vi "UHR-Fleezers Control (fpga) - avogadro 2.vi"() -> ()   [LabVIEW 2014]
doc: "UHR-Fleezers Instrument Control Code (fpga)"
uses:
  <vilib>/Platform/TimedLoop/XDataNode/timing_clust.ctl
  <vilib>/Platform/TimedLoop/XDataNode/nitl_modes.ctl
  <vilib>/Platform/TimedLoop/XDataNode/wakeup.ctl
  <vilib>/rvi/Emulation/niFpgaGetClockAttributes.vi
  <vilib>/rvi/Emulation/niFpgaSctlEmulationGetInTimedLoop.vi
  <vilib>/rvi/Emulation/niFpgaEmulationReportErrorSimple.vi
  <vilib>/rvi/Emulation/niFpgaProcessEmulError.vi
  <vilib>/rvi/eio/common/nirviEmuTemplateMethod_errors.vi
  <vilib>/rvi/interface/RandomDataEmulation/niFpgaRandomDataHandleErrors.vi
  <vilib>/rvi/Emulation/niFpgaCriticalErrorInLSC.vi
  <vilib>/eio/EIONode/EIONode.xnode
  <vilib>/eio/EIOMethodNode/EIOMethodNode.xnode
  <vilib>/rvi/DataTransferAndStorage/Container/XNode/niFpgaContainer.xnode
  <vilib>/rvi/interface/RandomDataEmulation/nirviRandomDataFpgaReadWriteTemplate.vi
  <vilib>/addons/control/pid/fpga.llb/XNode/niFpgaPID.xnode
  <vilib>/Platform/TimedLoop/XDataNode/XDataNode.xnode
  <vilib>/Platform/TimedLoop/XDataNode/XDNodeRunTimeDep.lvlib
panel:
  out "Tab Control":T1(tab)=enum."MCL trap control"
  in  "Set 3":bool
  in  "Set 2":bool=TRUE
  in  "Set 1":bool=TRUE
  in  "Trap Pos to FIFO":bool
  in  "N of AI1 Int Acq Sets":i16=2 min=1 max=3 step=1
  out "AI Late Counter":u8
  in  "ai count":u16=400
  in  "+ phase":bool
  in  "Phase count adjustment":i16
  out "Relative phase":i16
  in  "AI to FIFO":bool
  out "BD1 Frequency Out 1":u64
  out "BD1 Frequency Out 2":u64
  out "Trap Pos FIFO Timeout":u16
  out "Trap AI FIFO Timeout":u16
  in  "Trap FIFO Set Timeout":i32
  out "Tab Control 2":T2(tab)
  in  "Piezo offset Y points":u64
  in  "Piezo offset X points":u64
  in  "Piezo offset Xmin":u64
  in  "Piezo Offset Ymin":u64
  in  "Piezo Offset Increment":u64
  in  "Multiple trap 3 position offset \nfile":bool
  in  "FB output range":cluster{"output low":i16, "output high":i16}={"output low"=0, "output high"=3000}
  in  "FB Gains":T3={"proportional gain (Kc)"=10, "integral gain (Kc*Ts/Ti)"=5, "derivative gain (Kc*Td/Ts)"=0}
  in  "RD":bool
  in  "Swap F1 and F2":bool
  in  "Cont. Scan":bool
  in  "Abort scan":bool
  in  "Cycles per step":u64
  in  "Scan BD":bool
  in  "Number of scans":u16
  in  "Scan steps":u64
  in  "Scan freq.  increment":i64
  out "Scanning":bool
  in  "Start scan":bool
  in  "OSK Bd 1":bool
  in  "Reset Bd 1":bool
  in  "PMODE":bool
  in  "Direct RF Box \nCommunication":bool
  in  "Data BD 2":u8 format="%08b"
  in  "Data BD 1":u8 format="%08b"
  in  "Address":u8 format="%02x"
  in  "Update Data":bool
  in  "FPGA Controls\n RF Box":bool
  in  "Number Interlace Cycles":u8=2 min=1 max=3
  in  "Interlace Off Parameters":u8=1 min=1 max=3
  in  "Interlace ON/OFF":bool
  out "DIO Relative phase":i16
  in  "Phase count adjustment (DIO)":i16
  in  "+ phase (DIO)":bool
  out "DIO Late Counter":u8
  in  "DIO count 1 (ticks)":u16=400
  in  "DIO count 2 (ticks)":u16=400
  in  "DIO count 3 (ticks)":u16=400
  out "AI2 Y Sum Set 2":i16
  out "AI2 Y Sum Set 1":i16
  in  "FB Setpoint Set 1":i16 min=0 step=1
  in  "FB Reset Set 1":bool
  in  "FB On/Off Set 1":bool
  in  "FB Reset Set 2":bool
  in  "FB On/Off Set 2":bool
  in  "FB Setpoint Set 2":i16 min=0 step=1
  out "Scan I":u64
  in  "Amp switch delay":u8=5
  in  "BD 2 Amplitude 1":u16
  in  "BD 1 Amplitude 1":u16
  in  "BD 2 Frequency 1":u64
  in  "BD 1 Frequency 1":u64
  in  "BD 2 Amplitude 2":u16
  in  "BD 1 Amplitude 2":u16
  in  "BD 2 Frequency 2":u64
  in  "BD 1 Frequency 2":u64
  in  "BD 2 Amplitude 3":u16
  in  "BD 1 Amplitude 3":u16
  in  "BD 2 Frequency 3":u64
  in  "BD 1 Frequency 3":u64
  in  "BD 1 Delay (ticks)":u8
  in  "BD 2 Delay (Ticks)":u8 caption="Count(Ticks)"
  in  "Next trap write delay (ticks)":u8 caption="Count(Ticks)"
  out "Piezo X out":i16
  out "Piezo Y out":i16
  in  "Piezo Trap ON/Off (AO3)":i16
  in  "Piezo Trap X (AO5)":i16
  in  "Piezo Trap Y (AO4)":i16
  in  "Trap pos. FB Range":T4={"FB2 output low"=-1.0, "FB2 output high"=0.999969482421875}
  in  "FB Min frequency":u64
  in  "FB Max Frequency":u64
  in  "Dynamic Force FB (Ronen)":bool
  in  "Negate Diff?":bool
  in  "Diff FB Measurement?":bool
  in  "FB Trig Integrate":u32=1
  out "TTrig?":bool
  in  "TTrig Negate Pos":bool=TRUE
  out "Trap Pos FB Int Signal":fxp<+/-,24,9> format="%.18g"
  out "Trap Pos FB Int-Norm Signal":fxp<+/-,16,1> format="%.16g"
  in  "FPGA TTrig Thresh":i64
  in  "FPGA Trap Trig":bool
  out "Trap Pos FB Action":i64
  in  "Trap Pos. FB Offset Factor":i64
  in  "Trap Pos. FB Mult Factor":i64=2
  in  "Trap Pos. FB Reset":bool
  in  "Trap Pos FB Monitor T1 or T2":bool
  in  "AI1 X Scale":u16
  in  "Trap Pos FB Int Count":u16=100
  in  "Trap Pos FB Negate Action":bool
  out "AI1 X Set 2":fxp<+/-,16,1>
  out "AI1 X Set 1":fxp<+/-,16,1>
  in  "Trap Pos. FB SP":fxp<+/-,16,1>
  in  "Force feedback":bool
  out "TTrig Sig":i64
  out "TTrig Fin Thresh":i64
  in  "B factor":fxp<+/-,32,16>
  in  "Trap Pos. FB Gains":T5={"proportional gain (Kc)"=0.999969482421875, "integral gain (Kc*Ts/Ti)"=0.999969482421875, "derivative gain (Kc*Td/Ts)"=0.0}
  in  "ScanTrap 3 or Fl-laser":bool
  in  "1D or 2D Scan?":bool
  in  "Abort scan (MCL)":bool
  in  "MCL Scan Axis":bool
  in  "Cont. Scan (MCL)":bool
  out "Scan I (MCL)":u64
  in  "Number of scans (MCL)":u16
  out "Scanning MCL":bool
  in  "Scan steps (MCL)":u64
  in  "Cycles per step (MCL)":u64
  in  "Scan freq.  increment (MCL)":i16
  in  "Start scan (MCL)":bool
  in  "AO2 (X)":i16
  in  "AO1 (Y)":i16
  out "MCL Late Counter":u8
  in  "MCL count":u32=800
  out "MCL Relative Phase":i16
  in  "Phase count adjustment (MCL)":i16
  in  "+ phase (MCL)":bool
  out "APD2 int gate":bool
  out "APD3 out state":bool
  in  "APD Gate Operating Mode":u8 max=2 step=1
  in  "Invert APD Gate":bool
  in  "APD Gate OFF Count":u16=100
  in  "APD Gate ON Count":u16=300
  out "APD 1 Gate Late Counter":u8
  out "APD 1 Gate Relative Phase":i16
  in  "Phase count adjustment (APD 1 Gate)":i16
  in  "+ phase (APD 1 Gate)":bool
  out "APD 2 Counts 0":u32
  out "APD 2 Counts 1":u32
  out "APD 1 Counts 0":u32
  out "APD 1 Counts 1":u32
  out "APD1 out state":bool
  in  "APD AO scale factor":i16=1
  in  "APD to FIFO":bool
  in  "APD Acq Rate Count":u32=20000000
  out "APD Acq Late Counter":u8
  out "APD Acq Relative Phase":i16
  in  "Phase Count Adjustment (APD Acq)":i16
  in  "+ phase (APD Acq)":bool
  in  "Phase count adjustment (APD 2 Gate)":i16
  out "APD 2 Gate Late Counter":u8
  out "APD 2 Gate Relative Phase":i16
  in  "+ phase (APD 2 Gate)":bool
  out "APD2 out state":bool
  out "APD 3 Counts 0":u32
  out "APD 3 Counts 1":u32
  out "APD 3 Gate Late Counter":u8
  in  "Phase count adjustment (APD 3 Gate)":i16
  out "APD 3 Gate Relative Phase":i16
  in  "+ phase (APD 3 Gate)":bool
  out "APD1 int gate":bool
  out "APD3 int gate":bool
  in  "D3":i16
  in  "I3":i16=5
  in  "P3":i16=10
  in  "Green Filter Flipper":bool
  in  "Green FB Count":u16=1200
  out "Green Late Counter":u8
  out "Green FB Relative Phase":i16
  in  "Phase count adjustment (Green FB)":i16=10
  in  "+ phase (Green FB)":bool
  out "Green FB Sum":i16
  in  "Green int current ON count adj":u16=150
  in  "Current Out":u16=30000
  in  "Green FB On/Off":bool
  in  "Green FB Setpoint":i16=250 min=0 step=1
  in  "Green FB Reset":bool
  in  "Operating Mode 2":u8=2 max=2 step=1
  in  "Invert GI 2":bool
  in  "Green interlace OFF count 2":u16=900
  in  "Green interlace ON count 2":u16=300
  out "GI Late Counter 2":u8
  out "GI Relative phase 2":i16
  in  "Phase count adjustment (GI) 2":i16=20
  in  "+ phase (GI) 2":bool
  in  "Green interlace OFF count":u16=100
  out "GI Relative phase":i16
  in  "Phase count adjustment (GI)":i16
  in  "+ phase (GI)":bool
  in  "Green interlace ON count":u16=300
  out "GI Late Counter":u8
  in  "Invert GI":bool
  in  "Operating Mode":u8 max=2 step=1
  in  "+ phase (RI)":bool
  out "RI Relative phase":i16
  out "RI Late Counter":u8
  in  "Red interlace ON count":u16=300
  in  "Red interlace OFF count":u16=100
  in  "Invert RI":bool
  in  "Red Laser Operating Mode":u8 max=2 step=1
  in  "Phase count adjustment (RI)":i16
  out "Red FB Intensity":i16
  in  "RI Current Out":u16=30000
  in  "Red FB On/Off":bool
  in  "D4":i16
  in  "I4":i16=5
  in  "P4":i16=10
  in  "Red FB Setpoint":i16=250 min=0 step=1
  in  "Red FB Reset":bool
  in  "RI Operating Mode 2":u8=2 max=2 step=1
  in  "Invert RI 2":bool
  in  "Phase count adjustment (BI AO)":i16=20
  in  "Blue current ON count adj (AO)":u16=150
  in  "BI Current Out":i16=30000
  in  "Blue FB On/Off":bool
  in  "D5":i16
  in  "I5":i16=5
  in  "P5":i16=10
  in  "Blue FB Setpoint":i16=250 min=0 step=1
  in  "Blue FB Reset":bool
  in  "BI Operating Mode (AO)":u8=2 max=2 step=1
  in  "Invert BI (AO)":bool
  in  "Blue OFF count (AO)":u16=900
  in  "Blue ON count (AO)":u16=300
  out "BI Late Counter (AO)":u8
  out "BI Relative phase (AO)":i16
  in  "+ phase (BI AO)":bool
  in  "Phase count adjustment (BI D)":i16
  in  "Blue Laser Operating Mode (D)":u8 max=2 step=1
  in  "Invert BI (D)":bool
  in  "Blue interlace OFF count (D)":u16=100
  in  "Blue interlace ON count (D)":u16=300
  out "Blue Late Counter (D)":u8
  out "BI Relative phase (D)":i16
  in  "+ phase (BI D)":bool
  out "Blue Intensity":i16
  # "Only one of these can be on\nat a time:"
  # "Raster Scan AOD"
  # "1 (X)"
  # "2 (Y)"
  # "IR Intensity Feedback (RF BD 1)"
  # "False is usual, True is external loop method"
  # "Parameters if using the external RF switching loop"
  # "Parameters if using the usual internal RF switching method"
  # "FB Triggering Excitation Laser"
  # "Trap Pos. FB Gains"
  # "Trap Pos. FB Range"
  # "AO1 (Y)"
  # "2D"
  # "Trap 3"
  # "1D"
  # "Fl Laser"
  # "AO2 (X)"
  # "APD AO for aligning"
  # "Detection Loop"
  # "Green fluorescent laser digital gate interlacing loop"
  # "0 Forced ON\n1 Forced OFF\n2 Interlacing"
  # "Green FB Gains"
  # "Red fluorescent laser digital gate interlacing loop"
  # "Detection Loop"
  # "0 Forced ON\n1 Forced OFF\n2 Interlacing"
  # "Analog/FB Control Loop\n(Disabled)"
  # "Digital Control Loop"
  # "Blue laser intensity reading"
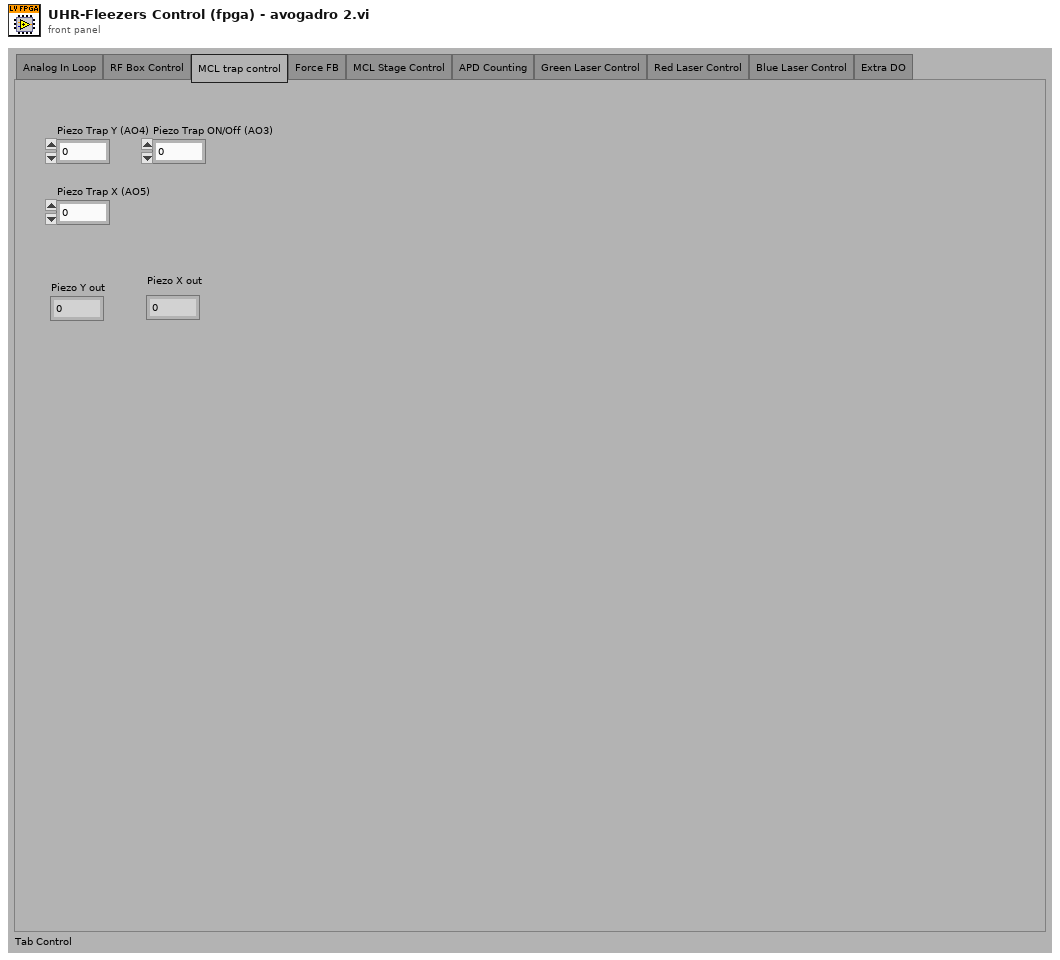
[diagram p1: front panel]
types:
  T1 = enum32{"Analog In Loop", "RF Box Control", "MCL trap control", "Force FB", "MCL Stage Control", "APD Counting", "Green Laser Control", "Red Laser Control", "Blue Laser Control", "Extra DO"}
  T2 = enum32{"Controls", "Interlacing Frequency and Amplitude Values", "Oscillate trap from memory"}
  T3 = cluster{"proportional gain (Kc)":i16, "integral gain (Kc*Ts/Ti)":i16, "derivative gain (Kc*Td/Ts)":i16}
  T4 = cluster{"FB2 output low":fxp<+/-,16,1>, "FB2 output high":fxp<+/-,16,1>}
  T5 = cluster{"proportional gain (Kc)":fxp<+/-,16,1>, "integral gain (Kc*Ts/Ti)":fxp<+/-,16,1>, "derivative gain (Kc*Td/Ts)":fxp<+/-,16,1>}
  T6 = typedef "XDNodeRunTimeDep.lvlib/timing_clust.ctl" = cluster{"Expected End [f-1]":u64, "Actual End [f-1]":u64, "Finished Late? [f-1]":bool, "Expected End [i-1]":u64, "Actual End [i-1]":u64, "Finished Late? [i-1]":bool, "Expected Start [i]":u64, "Actual Start [i]":u64, "Expected Start [f]":u64, "Actual Start [f]":u64, "Source Name":string, "Structure Name":string, "Period":i64, "Deadline":i64, "Offset":i64, "Start":i64, "Priority":i32, "Timeout":i32, "Mode":T7, "Wakeup Reason":T8, "Error":errorcluster, "Source Type":string, "Secondary Source Type":string, "Global End Time":u64, "Global Start Time":u64, "Frame Duration":u64, "Iteration Duration":u64, "Assigned CPU":i32, "I/O Scan Engine Mode":u32}
  T7 = typedef "XDNodeRunTimeDep.lvlib/nitl_modes.ctl" = enum32{"No Change", "Process missed periods, maintain original phase", "Discard missed periods, maintain original phase", "Process missed periods, ignore original phase", "Discard missed periods, ignore original phase"}
  T8 = typedef "XDNodeRunTimeDep.lvlib/wakeup.ctl" = enum32{"Normal", "Aborted", "Asynchronous wakeup", "Timing source error", "Timed loop error", "Timeout"}
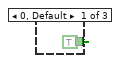
[diagram p2: hidden frame]
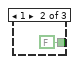
[diagram p3: hidden frame]
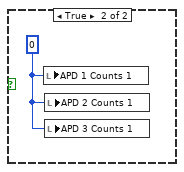
[diagram p5: hidden frame]
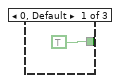
[diagram p7: hidden frame]
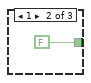
[diagram p8: hidden frame]
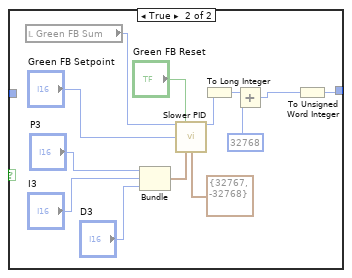
[diagram p11: hidden frame]
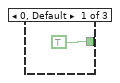
[diagram p12: hidden frame]
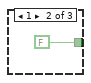
[diagram p13: hidden frame]
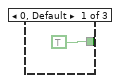
[diagram p14: hidden frame]
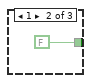
[diagram p15: hidden frame]
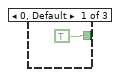
[diagram p17: hidden frame]
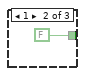
[diagram p18: hidden frame]
diagram:
  w1 = i16 0
  w6 = FALSE
  w4 = FALSE
  # "Control of MCL trap"
  # "timing array current index"
  # "timing array"
  # "timing counter (phase adjusted here)"
  # "late counter"
  n1 = flat-sequence "FPGA initialization to do before running any of the loops" {
    tunnel: [u16 0 ("DIO count 3 (ticks)")] -> w2
    tunnel: [w14] -> _
    frame #0 {
      w13 = FALSE ("Enable")
      # "BD 2 (Y)"
      # "BD 1 (X)"
      # "Start up expansion chassis early\nto avoid delays later"
      # "This pin controls udclk on the RF boards.\nWhen initially configuring the boards, this pin needs to be\nconfigured as a high impedance input.  Later it will be switched\nto an output."
      # "Initial setting of DIO data and \naddress to low (before reset).  \nThis needs to happen before the other\ncontrol method loops execute."
      n2 = xnode "FPGA I/O Node"("Chassis2/Mod1/AO0"=u16 0 ("Chassis2/Mod4/AO0")) -> ("Chassis2/Mod2/AI0"=w14:i16)  [unwired: 2 in, 2 out]
      n3 = xnode "FPGA I/O Method Node"("Enable"=w13) -> ()  [unwired: 1 in, 1 out]
      n4 = xnode "FPGA I/O Method Node"("Enable"=w13) -> ()  [unwired: 1 in, 1 out]
      n5 = xnode "FPGA I/O Node"("Connector1/DIO0"=FALSE, "Connector1/DIO1"=FALSE, "Connector1/DIO2"=FALSE, "Connector1/DIO3"=FALSE, "Connector1/DIO4"=FALSE, "Connector1/DIO5"=FALSE, "Connector1/DIO6"=FALSE, "Connector1/DIO7"=FALSE, "Connector1/DIO8"=FALSE, "Connector1/DIO9"=FALSE, "Connector1/DIO10"=FALSE, "Connector1/DIO11"=FALSE, "Connector1/DIO12"=FALSE, "Connector1/DIO13"=FALSE, "Connector1/DIO15"=FALSE, "Connector1/DIO20"=FALSE, "Connector1/DIO21"=FALSE, "Connector1/DIO22"=FALSE, "Connector1/DIO23"=FALSE, "Connector1/DIO24"=FALSE, "Connector1/DIO25"=FALSE, "Connector1/DIO26"=FALSE, "Connector1/DIO27"=FALSE, "Connector1/DIO14"=FALSE) -> ()  [unwired: 24 in, 24 out]
    }
  }
  n6 = local read "AO1 (Y)"() -> (w11:i16)
  n7 = local read "AO2 (X)"() -> (w10:i16)
  n8 = node-c288() -> (w9:T6)  [unwired: 1 in]
  n9 = To Unsigned Long Integer(number=w2) -> (unsigned 32bit integer=w7:u32)
  n10 = timed-loop "RF box board DIO control: control bits" {
    timing: w9 -> [_]
    timing-out: [_] -> w8
    tunnel: [w43] -> _
    tunnel: w2 -> [w43]
    stop <- FALSE stop-if-true
    n11 = xnode "FPGA I/O Node"("Connector1/DIO16"="RD", "Connector1/DIO17"="PMODE", "Connector1/DIO18"="OSK Bd 1", "Connector1/DIO19"="Reset Bd 1", "Connector0/DIO3"="Green Filter Flipper") -> ()  [unwired: 5 in, 5 out]
  }
  n12 = while "RF box board DIO control: parallel communication" {
    shift-right: [w58] -> _
    shift-left: w2 -> [w57]
    shift-right: [w56] -> _
    shift-left: FALSE ("Swap F1 and F2") -> [w55]
    shift-right: [w50] -> _
    shift-left: u64 0 -> [w51]
    stop <- FALSE stop-if-true
    n13 = flat-sequence {
      tunnel: w55 -> [w62]
      tunnel: w57 -> [w60]
      tunnel: [w62] -> w54
      tunnel: [w61] -> w53
      tunnel: [w60] -> w52
      tunnel: [w70] -> w58
      tunnel: [w69] -> w56
      tunnel: w54 -> [w68]
      tunnel: w53 -> [w66]
      tunnel: w52 -> [w65]
      tunnel: w51 -> [w64]
      tunnel: [w63] -> w50
      frame #0 {
        n14 = call "Loop Timer"("Count(Ticks)"=w60) -> ("Tick Count(Ticks)"=w61:u16)
      }
      frame #1 {
        n15 = flat-sequence {
          tunnel: ["FPGA Controls\n RF Box"] -> w67
          tunnel: w68 -> [w71]
          tunnel: [w123] -> w70
          tunnel: [w136] -> w69
          tunnel: w67 -> [w135]
          tunnel: w66 -> [w129]
          tunnel: w65 -> [w126]
          tunnel: w64 -> [w101]
          tunnel: [w100] -> w63
          frame #0 {
            n16 = case shown="True" "FPGA Controls\n RF Box" {
              tunnel: w71 -> [_ w73]
              frame False {
              }
              frame True {
                n17 = flat-sequence {
                  tunnel: w73 -> [w83]
                  frame #0 {
                    n18 = First Call?() -> (First Call?: T/F=w74:bool)
                    n19 = case shown="True" w74 {
                      frame False {
                      }
                      frame True {
                        # "BD 2"
                        # "BD 1"
                        # "If first time data updated, be sure to set WR high and UDCLK low\nbefore setting data and address bits."
                        n20 = xnode "FPGA I/O Method Node"("Enable"=TRUE) -> ("FPGA I/O Out"=w76:refnum<k21>)  [unwired: 1 in]
                        n21 = xnode "FPGA I/O Method Node"("Enable"=TRUE) -> ("FPGA I/O Out"=w79:refnum<k21>)  [unwired: 1 in]
                        n22 = xnode "FPGA I/O Node"("Connector1/DIO15"=TRUE) -> ()  [unwired: 1 in, 1 out]
                        n23 = xnode "FPGA I/O Node"("I/O Item"=FALSE ("Connector1/DIO30"), "FPGA I/O In"=w76) -> ()  [unwired: 1 out]
                        n24 = xnode "FPGA I/O Node"("I/O Item"=FALSE ("Connector1/DIO30"), "FPGA I/O In"=w79) -> ()  [unwired: 1 out]
                      }
                    }
                  }
                  frame #1 {
                    n25 = case shown="False" FALSE {
                      tunnel: w83 -> [w85 _]
                      frame False {
                        # "Usual operation"
                        n26 = disable-structure shown="Disabled" {
                          disable-tunnel: w85 -> [w87 _]
                          disable-tunnel: "Amp switch delay" -> [w86 _]
                          frame Disabled {
                            n27 = flat-sequence "BD 2 (Y)" {
                              tunnel: w87 -> [w89]
                              tunnel: w86 -> [w90]
                              frame #0 {
                                n28 = call "Wait7"("Count(Ticks)"="BD 2 Delay (Ticks)") -> ()  [unwired: 1 out]
                              }
                              frame #1 {
                                # "switch frequency"
                                n29 = xnode "FPGA I/O Node"("Connector1/DIO37"=w89) -> ()  [unwired: 1 in, 1 out]
                              }
                              frame #2 {
                                # "~5 ticks is usual"
                                n30 = call "Wait5"("Count(Ticks)"=w90) -> ()  [unwired: 1 out]
                              }
                              frame #3 {
                                # "this switches amplitude"
                                # "switch amplitude"
                                # "send udclk high"
                                n31 = xnode "FPGA I/O Node"("Connector1/DIO29"=TRUE ("Connector1/DIO15")) -> ()  [unwired: 1 in, 1 out]
                              }
                              frame #4 {
                                # "reset to be ready for next\ncycle"
                                # "send udclk low"
                                n32 = xnode "FPGA I/O Node"("Connector1/DIO29"=FALSE ("Connector1/DIO15")) -> ()  [unwired: 1 in, 1 out]
                              }
                            }
                          }
                          frame Enabled {
                          }
                        }
                        n33 = flat-sequence "BD 1 (X)" {
                          tunnel: w85 -> [w94]
                          tunnel: "Amp switch delay" -> [w95]
                          frame #0 {
                            n34 = call "Wait6"("Count(Ticks)"="BD 1 Delay (ticks)") -> ()  [unwired: 1 out]
                          }
                          frame #1 {
                            # "switch frequency"
                            n35 = xnode "FPGA I/O Node"("Connector1/DIO36"=w94) -> ()  [unwired: 1 in, 1 out]
                          }
                          frame #2 {
                            # "~5 ticks is usual"
                            n36 = call "Wait4"("Count(Ticks)"=w95) -> ()  [unwired: 1 out]
                          }
                          frame #3 {
                            # "this switches amplitude"
                            # "switch amplitude"
                            # "send udclk high"
                            n37 = xnode "FPGA I/O Node"("Connector1/DIO30"=TRUE ("Connector1/DIO15")) -> ()  [unwired: 1 in, 1 out]
                          }
                          frame #4 {
                            # "reset to be ready for next\ncycle"
                            # "send udclk low"
                            n38 = xnode "FPGA I/O Node"("Connector1/DIO30"=FALSE ("Connector1/DIO15")) -> ()  [unwired: 1 in, 1 out]
                          }
                        }
                      }
                      frame True {
                        # "Operation when you need a long delay for either X or Y to synchonize AOD light out phase (> ~100 ticks)."
                        # "Trigger the external loop by sending the boolean FSK value through a FIFO"
                      }
                    }
                  }
                  frame #2 {
                  }
                }
              }
            }
          }
          frame #1 {
            # "This is the prior cycle's on time"
            # "increment timing\nindex, reset to 0 if \nend of matrix"
            # "Reset to begginning (1) when number of cycles reached."
            # "timing index"
            # "build byte stacks for writing data\n(must correspond to addresses array constant)"
            # "Timing housekeeping"
            # "Adjust phase if late\n(maintains constant phase relationship between cycles)"
            n39 = feedback #1(u8 0 ("t")) -> (w132:u8)
            n40 = Increment(x=w132) -> (x+1=w175:u8)
            n41 = Increment(x="Number Interlace Cycles") -> (x+1=w170:u8)
            n42 = Equal?(x=w175, y=w170) -> (x = y?=w177:bool)
            n43 = Select(t=u8 1, s=w177, f=w175) -> (s? t:f=w131:u8)
            n44 = feedback-in #1(w131) -> ()
            n45 = Increment(x=w131) -> (x+1=w172:u8)
            n46 = Equal?(x=w172, y=w170) -> (x = y?=w173:bool)
            n47 = Select(t=u8 1, s=w173, f=w172) -> (s? t:f=w169:u8)
            n48 = Select(t=w169, s="Interlace ON/OFF", f="Interlace Off Parameters") -> (s? t:f=w102:u8)
            n49 = case shown="1, Default" w102 {
              tunnel: [w222 w432 "BD 1 Frequency 3"] -> w165
              tunnel: [w265 "BD 2 Frequency 2" "BD 2 Frequency 3"] -> w154
              tunnel: ["BD 2 Amplitude 1" "BD 2 Amplitude 2" "BD 2 Amplitude 3"] -> w111
              tunnel: [w231 w430 "BD 1 Amplitude 3"] -> w114
              tunnel: "FB output range" -> [w235 w427 _]
              tunnel: w101 -> [w230 w429 w445]
              tunnel: [w222 w429 w445] -> w100
              tunnel: "FB Gains" -> [w217 w428 _]
              frame 1, Default {
                w249 = fxp<+/-,24,9> 0.0 ("AI1 X Set 2")
                w243 = u16 0
                w261 = u64 0 ("f")
                # "Explanation of raster scanning:\n1. Cycles: increment counter by 1 every time interlace cycle returns to trap 1. As long as \n  Cycle per Step is larger than counter, keep incrementing counter and do not change step counter.\n  Once counter is equal to Cycles per step, zero counter and increment step counter.\n2. Steps: Increments up every time cycles counter equals cycles per step. Performs the following:\n- To determine DIRECTION of frequency change:  If ScanstepX2 is EQUAL to step counter (full for-back scan finished)\n   frequency increment is set to zero, AND step counter is set to zero. \n   Otherwise: if no change to step counter (because cycleperstep>cycle counter), then no change to frequency\n   increment. \n   If step counter has changed (cycleperstep=cycle counter), then need to figure out direction of frequency change:\n   if step counter is EQUAL to Scansteps: No change to frequency increment\n   Otherwise: If scan steps > step counter - 1 (forward scan NOT completed): increment frequency by 1\n                       If scan steps equal or smaller than step counter -1 (forward scan completed): increment frequency by -1\n\n3. Scans: Increment scan counter every time step counter equals 2Xscan steps (full for-back scan completed)\n    if number of scans > scan counter: Send TRUE to scanning, continue scan\n    if number of scans = scan counter: Send FALSE to Scanning, Scan finished.\n\n  The wire with the asterik can be used as the index for getting the mirror positions in the offset scan."
                # "Added by Ronen -\nUpper and Lower \nLimits for the FB \ngenerated frequency\nto avoid losing bead \nwhen tether breaks"
                # "Changed by Ronen - correction \nby PID is now implemented not on \nthe Base BD1 frequency but on the last\nfrequency sent."
                # "BD1 Amp 1"
                # "This signal integration happens no matter what\nso that correct setpoints can be chosen before \nturning on the FB."
                # "Trap 1"
                n50 = local read "AI1 X Set 2"() -> (w225:fxp<+/-,16,1>)
                n51 = local read "AI1 X Set 1"() -> (w246:fxp<+/-,16,1>)
                n52 = local read "Scanning"() -> (w266:bool)
                n53 = Multiply(x=w225, y="B factor") -> (x*y=w223:fxp<+/-,48,17>)
                n54 = Or(x=w266, y="Start scan") -> (x .or. y?=w259:bool)
                n55 = case shown="True" "Diff FB Measurement?" {
                  tunnel: w223 -> [w284 w293]
                  tunnel: w246 -> [w283 w294]
                  tunnel: [w281 w285] -> w247
                  frame False {
                    n56 = Select(t=w283, s="Trap Pos FB Monitor T1 or T2", f=w284) -> (s? t:f=w281:fxp<+/-,48,17>)
                  }
                  frame True {
                    n57 = Subtract(x=w294, y=w293) -> (x-y=w286:fxp<+/-,48,17>)
                    n58 = Not(x="Negate Diff?") -> (.not. x?=w292:bool)
                    n59 = Boolean To (0,1)(Boolean="Negate Diff?") -> (0, 1=w290:i16)
                    n60 = Boolean To (0,1)(Boolean=w292) -> (0, 1=w291:i16)
                    n61 = Negate(x=w290) -> (-x=w289:i16)
                    n62 = Add(x=w289, y=w291) -> (x+y=w287:i16)
                    n63 = Multiply(x=w287, y=w286) -> (x*y=w285:fxp<+/-,63,32>)
                  }
                }
                n64 = Not(x="Abort scan") -> (.not. x?=w257:bool)
                n65 = And(x=w257, y=w259) -> (x .and. y?=w256:bool)
                n66 = case "For raster scanning" shown="True" w256 {
                  tunnel: [u64 0 w417] -> w262
                  tunnel: "Start scan" -> [_ w402]
                  tunnel: [u64 1 w379] -> w216
                  frame False {
                    n67 = local write "Scanning"(FALSE ("scanning")) -> ()
                  }
                  frame True {
                    w387 = i64 0
                    w386 = u64 0
                    # "scan incr."
                    # "freq. incr. mult."
                    # "count steps"
                    # "count number of cycles"
                    n68 = feedback #2(w386) -> (w414:u64)
                    n69 = Select(t=w386, s=w402, f=w414) -> (s? t:f=w416:u64)
                    n70 = Increment(x=w416) -> (x+1=w413:u64)
                    n71 = Greater?(x="Cycles per step", y=w413) -> (0:w396:bool)
                    n72 = Select(t=w413, s=w396, f=w386) -> (s? t:f=w412:u64)
                    n73 = feedback-in #2(w412) -> ()
                    n74 = feedback #3(w386) -> (w411:u64)
                    n75 = Select(t=w386, s=w402, f=w411) -> (s? t:f=w406:u64)
                    n76 = Increment(x=w406) -> (x+1=w410:u64)
                    n77 = Add(x="Scan steps", y="Scan steps") -> (x+y=w409:u64)
                    n78 = Select(t=w406, s=w396, f=w410) -> (s? t:f=w391:u64)
                    n79 = Greater?(x=w409, y=w391) -> (0:w390:bool)
                    n80 = Select(t=w391, s=w390, f=w386) -> (s? t:f=w407:u64)
                    n81 = feedback-in #3(w407) -> ()
                    n82 = Equal?(x="Scan steps", y=w391) -> (x = y?=w395:bool)
                    n83 = Greater?(x="Scan steps", y=w406) -> (0:w405:bool)
                    n84 = feedback #4(w387) -> (w408:i64)
                    n85 = Select(t=w387, s=w402, f=w408) -> (s? t:f=w393:i64)
                    n86 = Increment(x=w393) -> (x+1=w404:i64)
                    n87 = Decrement(x=w393) -> (x-1=w403:i64)
                    n88 = Select(t=w404, s=w405, f=w403) -> (s? t:f=w394:i64)
                    n89 = Select(t=w393, s=w395, f=w394) -> (s? t:f=w392:i64)
                    n90 = Select(t=w393, s=w396, f=w392) -> (s? t:f=w388:i64)
                    n91 = Select(t=w388, s=w390, f=w387) -> (s? t:f=w389:i64)
                    n92 = feedback-in #4(w389) -> ()
                    n93 = feedback #5(w386) -> (w401:u64)
                    n94 = Select(t=w386, s=w402, f=w401) -> (s? t:f=w397:u64)
                    n95 = Increment(x=w397) -> (x+1=w398:u64)
                    n96 = Select(t=w397, s=w390, f=w398) -> (s? t:f=w380:u64)
                    n97 = Greater?(x="Number of scans", y=w380) -> (0:w383:bool)
                    n98 = Multiply(x="Scan freq.  increment", y=w393) -> (x*y=w417:i64)
                    n99 = Select(t=TRUE, s="Cont. Scan", f=w383) -> (s? t:f=w382:bool)
                    "Scanning" <- w382
                    n100 = Select(t=w380, s=w382, f=w386) -> (s? t:f=w399:u64)
                    n101 = feedback-in #5(w399) -> ()
                    n102 = Increment(x=w380) -> (x+1=w379:u64)
                  }
                }
                "Scan I" <- w216
                n103 = feedback #6(w243) -> (w242:u16)
                n104 = Increment(x=w242) -> (x+1=w244:u16)
                n105 = Greater Or Equal?(x=w244, y="Trap Pos FB Int Count") -> (x >= y?=w229:bool)
                n106 = Select(t=w243, s=w229, f=w244) -> (s? t:f=w245:u16)
                n107 = feedback-in #6(w245) -> ()
                n108 = feedback #7(w249) -> (w248:fxp<+/-,24,9>)
                n109 = Add(x=w247, y=w248) -> (x+y=w241:fxp<+/-,24,9>)
                n110 = case "For intensity feedback" shown="True" "FB On/Off Set 1" {
                  tunnel: [w419 w425] -> w231
                  tunnel: w235 -> [_ w426]
                  tunnel: "BD 1 Amplitude 1" -> [w419 _]
                  tunnel: w217 -> [_ w420]
                  frame False {
                  }
                  frame True {
                    n111 = local read "AI2 Y Sum Set 1"() -> (w423:i16)
                    n112 = call "Slower PID.vi"("process variable"=w423, "reset?"="FB Reset Set 1", "setpoint"="FB Setpoint Set 1", "PID gains (x 2^8)"=w420, "output range"=w426) -> ("output"=w421:i16)  [unwired: 10 out]
                    n113 = To Unsigned Word Integer(number=w421) -> (unsigned 16bit integer=w425:u16)
                  }
                }
                n114 = Select(t=w249, s=w229, f=w241) -> (s? t:f=w252:fxp<+/-,24,9>)
                n115 = feedback-in #7(w252) -> ()
                n116 = Divide(x=w241, y="Trap Pos FB Int Count") -> (x/y=w236:fxp<+/-,16,1>)
                n117 = feedback #8(fxp<+/-,24,9> 0.0 ("AI1 X Set 2")) -> (w253:fxp<+/-,24,9>)
                n118 = Select(t=w241, s=w229, f=w253) -> (s? t:f=w254:fxp<+/-,24,9>)
                "Trap Pos FB Int Signal" <- w254
                n119 = feedback-in #8(w254) -> ()
                n120 = feedback #9(fxp<+/-,16,1> 0.0 ("Trap Pos FB Int-Norm Signal")) -> (w238:fxp<+/-,16,1>)
                n121 = Select(t=w236, s=w229, f=w238) -> (s? t:f=w237:fxp<+/-,16,1>)
                "Trap Pos FB Int-Norm Signal" <- w237
                n122 = feedback-in #9(w237) -> ()
                n123 = case "For position feedback" shown="True" "Force feedback" {
                  tunnel: [i64 0 w300] -> w234
                  tunnel: w236 -> [_ w297]
                  tunnel: w229 -> [_ w296]
                  frame False {
                  }
                  frame True {
                    n124 = feedback #10(i64 0) -> (w299:i64)
                    n125 = case shown="False" w296 {
                      tunnel: [w301 w305] -> w300
                      tunnel: w299 -> [w301 _]
                      tunnel: w297 -> [_ w304]
                      frame False {
                      }
                      frame True {
                        n126 = xnode ("PID")("process variable"=w304, "reset?"="Trap Pos. FB Reset", "setpoint"="Trap Pos. FB SP", "PID gains"="Trap Pos. FB Gains", "output range"="Trap pos. FB Range") -> ("output"=w314:fxp<+/-,16,1>)
                        n127 = Negate(x=w314) -> (-x=w313:fxp<+/-,17,2>)
                        n128 = Select(t=w313, s="Trap Pos FB Negate Action", f=w314) -> (s? t:f=w310:fxp<+/-,17,2>)
                        n129 = Scale By Power Of 2(n=u32 15, x=u32 1) -> (x*2^n=w307:u32)
                        n130 = Multiply(x=w310, y=w307) -> (x*y=w306:fxp<+/-,17,17>)
                        n131 = To Quad Integer(1:w306) -> (0:w318:i64)
                        "Trap Pos FB Action" <- w318
                        n132 = Multiply(x=w318, y="Trap Pos. FB Mult Factor") -> (x*y=w316:i64)
                        n133 = Add(x=w316, y="Trap Pos. FB Offset Factor") -> (x+y=w305:i64)
                        n134 = disable-structure shown="Disabled" {
                          disable-tunnel: w305 -> [w325 _]
                          frame Disabled {
                            w329 = u32 0
                            n135 = feedback #11() -> (w326:i64)  [unwired: 1 in]
                            n136 = Add(x=w325, y=w326) -> (x+y=w323:i64)
                            n137 = feedback #12(w329) -> (w331:u32)
                            n138 = Increment(x=w331) -> (x+1=w320:u32)
                            n139 = Greater Or Equal?(x=w320, y="FB Trig Integrate") -> (x >= y?=w321:bool)
                            n140 = Select(t=i64 0, s=w321, f=w323) -> (s? t:f=w327:i64)
                            n141 = feedback-in #11(w327) -> ()
                            n142 = Select(t=w329, s=w321, f=w320) -> (s? t:f=w330:u32)
                            n143 = feedback-in #12(w330) -> ()
                            n144 = And(x=w321, y="FPGA Trap Trig") -> (x .and. y?=w328:bool)
                            n145 = case "Trap FB trigger excitation laser ON" shown="True" w328 {
                              tunnel: w323 -> [_ w335]
                              tunnel: w320 -> [_ w333]
                              frame False {
                              }
                              frame True {
                                n146 = Not(x="TTrig Negate Pos") -> (.not. x?=w342:bool)
                                n147 = Boolean To (0,1)(Boolean="TTrig Negate Pos") -> (0, 1=w340:i16)
                                n148 = Boolean To (0,1)(Boolean=w342) -> (0, 1=w341:i16)
                                n149 = Negate(x=w340) -> (-x=w339:i16)
                                n150 = Add(x=w339, y=w341) -> (x+y=w338:i16)
                                n151 = Multiply(x=w338, y=w335) -> (x*y=w337:i64)
                                "TTrig Sig" <- w337
                                n152 = Multiply(x="FPGA TTrig Thresh", y=w333) -> (x*y=w334:i64)
                                "TTrig Fin Thresh" <- w334
                                n153 = Greater Or Equal?(x=w337, y=w334) -> (x >= y?=w336:bool)
                                n154 = case shown="True" w336 {
                                frame False {
                                }
                                frame True {
                                w345 = TRUE ("Green FB On/Off")
                                w347 = u8 2 ("Operating Mode")
                                n155 = local write "Operating Mode 2"(w347) -> ()
                                n156 = local write "Operating Mode"(w347) -> ()
                                n157 = local write "Green FB On/Off"(w345) -> ()
                                n158 = local write "FPGA Trap Trig"(FALSE ("FPGA Trap Trig")) -> ()
                                "TTrig?" <- w345
                                }
                                }
                              }
                            }
                          }
                          frame Enabled {
                          }
                        }
                      }
                    }
                    n159 = feedback-in #10(w300) -> ()
                  }
                }
                n160 = And(x="Force feedback", y="Dynamic Force FB (Ronen)") -> (x .and. y?=w219:bool)
                n161 = case shown="False" w219 {
                  tunnel: w234 -> [w272 w276]
                  tunnel: [w271 w275] -> w232
                  tunnel: w230 -> [_ w274]
                  tunnel: w229 -> [_ w273]
                  frame False {
                    # "(BD1 Frequency 1)"
                    n162 = Add(x="BD 1 Frequency 1", y=w272) -> (x+y=w271:u64)
                  }
                  frame True {
                    n163 = case shown="False" w273 {
                      tunnel: w276 -> [_ w280]
                      tunnel: [w277 w279] -> w275
                      tunnel: w274 -> [w277 w278]
                      frame False {
                      }
                      frame True {
                        n164 = Add(x=w278, y=w280) -> (x+y=w279:u64)
                      }
                    }
                  }
                }
                n165 = Select(t=w261, s="Scan BD", f=w262) -> (s? t:f=w260:u64)
                n166 = Select(t=w262, s="Scan BD", f=w261) -> (s? t:f=w263:u64)
                n167 = Add(x=w260, y="BD 2 Frequency 1") -> (x+y=w265:u64)
                n168 = Compound Arithmetic op=ADD(i64 0 ("f"), w232, w263) -> (w228:u64)
                n169 = In Range and Coerce(upper limit="FB Max Frequency", x=w228, lower limit="FB Min frequency") -> (coerced(x)=w222:u64)  [unwired: 1 out]
                "BD1 Frequency Out 1" <- w222
              }
              frame 2 {
                # "Trap 2"
                n170 = case shown="True" "FB On/Off Set 2" {
                  tunnel: ["BD 1 Amplitude 2" w440] -> w430
                  tunnel: w427 -> [_ w441]
                  tunnel: w428 -> [_ w438]
                  frame False {
                  }
                  frame True {
                    n171 = local read "AI2 Y Sum Set 2"() -> (w443:i16)
                    n172 = call "Slower PID.vi"("process variable"=w443, "reset?"="FB Reset Set 2", "setpoint"="FB Setpoint Set 2", "PID gains (x 2^8)"=w438, "output range"=w441) -> ("output"=w439:i16)  [unwired: 10 out]
                    n173 = To Unsigned Word Integer(number=w439) -> (unsigned 16bit integer=w440:u16)
                  }
                }
                n174 = Add(x="BD 1 Frequency 2", y=i64 0 ("f")) -> (x+y=w432:u64)
                "BD1 Frequency Out 2" <- w432
              }
              frame 3 {
                # "Fluorescence period"
              }
            }
            n175 = feedback-in #13(w129) -> ()
            n176 = feedback #13(w129) -> (w128:u16)
            n177 = Select(t=w131, s="Interlace ON/OFF", f="Interlace Off Parameters") -> (s? t:f=w168:u8)
            n178 = Subtract(x=w129, y=w128) -> (x-y=w127:u16)
            n179 = Subtract "The error"(x=w127, y=w126) -> (x-y=w104:u16)
            n180 = case shown="1, Default" w168 {
              tunnel: ["DIO count 1 (ticks)" "DIO count 2 (ticks)" "DIO count 3 (ticks)"] -> w125
              frame 1, Default {
              }
              frame 2 {
              }
              frame 3 {
              }
            }
            n181 = Number To Boolean Array(number=w104) -> (Boolean array=w105:bool[])
            n182 = Or Array Elements(Boolean array=w105) -> (logical OR=w103:bool)
            n183 = Boolean To (0,1)(Boolean=w103) -> (0, 1=w110:i16)
            n184 = To Unsigned Byte Integer(number=w110) -> (unsigned 8bit integer=w107:u8)
            n185 = feedback #14(u8 0) -> (w108:u8)
            n186 = Add(x=w107, y=w108) -> (x+y=w106:u8)
            "DIO Late Counter" <- w106
            n187 = feedback-in #14(w106) -> ()
            n188 = Subtract(x=w125, y=w104) -> (x-y=w124:u16)
            n189 = Split Number(x=w165) -> (hi(x)=w164:u32, lo(x)=w163:u32)
            n190 = Split Number(x=w154) -> (hi(x)=w159:u32, lo(x)=w158:u32)
            n191 = Boolean To (0,1)(Boolean="+ phase (DIO)") -> (0, 1=w121:i16)
            n192 = Split Number(x=w164) -> (lo(x)=w162:u16)  [unwired: 1 out]
            n193 = Split Number(x=w163) -> (hi(x)=w161:u16, lo(x)=w160:u16)
            n194 = Split Number(x=w159) -> (lo(x)=w157:u16)  [unwired: 1 out]
            n195 = Split Number(x=w158) -> (hi(x)=w156:u16, lo(x)=w155:u16)
            n196 = Split Number(x=w114) -> (hi(x)=w116:u8, lo(x)=w115:u8)
            n197 = Split Number(x=w111) -> (hi(x)=w113:u8, lo(x)=w112:u8)
            n198 = Split Number(x=w162) -> (hi(x)=w153:u8, lo(x)=w152:u8)
            n199 = Split Number(x=w161) -> (hi(x)=w151:u8, lo(x)=w150:u8)
            n200 = Split Number(x=w157) -> (hi(x)=w146:u8, lo(x)=w145:u8)
            n201 = Split Number(x=w160) -> (hi(x)=w149:u8, lo(x)=w148:u8)
            n202 = Split Number(x=w156) -> (hi(x)=w144:u8, lo(x)=w143:u8)
            n203 = Split Number(x=w155) -> (hi(x)=w142:u8, lo(x)=w141:u8)
            n204 = Multiply(x=w121, y="Phase count adjustment (DIO)") -> (x*y=w117:i16)
            n205 = feedback #15(i16 0) -> (w119:i16)
            n206 = Subtract(x=w119, y=w117) -> (x-y=w118:i16)
            "DIO Relative phase" <- w118
            n207 = feedback-in #15(w118) -> ()
            n208 = Add(x=w124, y=w117) -> (x+y=w123:u16)
            n209 = Build Array "BD 1 A Stack"(w116, w115) -> (w138:u8[])
            n210 = Build Array "BD 2 A Stack"(w113, w112) -> (w137:u8[])
            n211 = Build Array "BD 1 nu Stack"(w153, w152, w151, w150, w149, w148) -> (w147:u8[])
            n212 = Build Array "BD 2 nu Stack"(w146, w145, w144, w143, w142, w141) -> (w140:u8[])
            n213 = case shown="2" w102 {
              tunnel: [w208 w211] -> w136
              tunnel: [u8 10 u8 4] -> w139
              tunnel: "Swap F1 and F2" -> [w209 w211]
              frame 2 {
                # "F2"
                n214 = Not(x=w209) -> (.not. x?=w208:bool)
              }
              frame 1, Default {
                # "low chooses F1"
                # "F1"
              }
            }
            n215 = case "If FPGA is controlling (toggling) RF synth" shown="True" w135 {
              tunnel: w147 -> [_ w184]
              tunnel: w140 -> [_ w183]
              tunnel: w139 -> [_ w182]
              tunnel: w138 -> [_ w181]
              tunnel: w137 -> [_ w180]
              frame False {
              }
              frame True {
                # "Write next amp.\n(wait until beginning of next loop iteration to update)"
                n216 = flat-sequence "Update the next F1 and F2 frequency value (the actual frequency won't change until FSK is switched).\nThen load the next amplitude value into buffer, but don't update it until the next cycle." {
                  tunnel: w183 -> [w186]
                  tunnel: w184 -> [w187]
                  tunnel: [w187] -> w179
                  tunnel: [w186] -> w178
                  tunnel: w182 -> [w188]
                  tunnel: w179 -> [w190]
                  tunnel: w178 -> [w189]
                  tunnel: w181 -> [w201]
                  tunnel: w180 -> [w200]
                  frame #0 {
                    # "To possibly send\nthese writes to very\nend of loop (for x and\ny phase adjust)"
                    n217 = call "Wait8"("Count(Ticks)"="Next trap write delay (ticks)") -> ()  [unwired: 1 out]
                  }
                  frame #1 {
                    n218 = for {
                      tunnel: w190 -> [w196] mode=indexing
                      tunnel: w189 -> [w195] mode=indexing
                      tunnel: w188 -> [w193]
                      i -> [w194]
                      # "Write next freq."
                      n219 = To Unsigned Byte Integer(number=w194) -> (unsigned 8bit integer=w191:u8)
                      n220 = Add(x=w193, y=w191) -> (x+y=w192:u8)
                      n221 = call "write to RF synth bd.vi"("Address Byte"=w192, "BD 2 Byte"=w195, "BD 1 Byte"=w196) -> ()
                    }
                  }
                  frame #2 {
                    w197 = TRUE ("Connector1/DIO15")
                    # "send udclk high\n(BD 1 and 2)"
                    n222 = xnode "FPGA I/O Node"("Connector1/DIO30"=w197, "Connector1/DIO29"=w197) -> ()  [unwired: 2 in, 2 out]
                  }
                  frame #3 {
                    w198 = FALSE ("Connector1/DIO15")
                    n223 = xnode "FPGA I/O Node"("Connector1/DIO30"=w198, "Connector1/DIO29"=w198) -> ()  [unwired: 2 in, 2 out]
                  }
                  frame #4 {
                    n224 = for {
                      tunnel: w201 -> [w207] mode=indexing
                      tunnel: w200 -> [w206] mode=indexing
                      tunnel: u8 33 -> [w204]
                      i -> [w205]
                      n225 = To Unsigned Byte Integer(number=w205) -> (unsigned 8bit integer=w202:u8)
                      n226 = Add(x=w204, y=w202) -> (x+y=w203:u8)
                      n227 = call "write to RF synth bd.vi"("Address Byte"=w203, "BD 2 Byte"=w206, "BD 1 Byte"=w207) -> ()
                    }
                  }
                }
              }
            }
          }
        }
      }
    }
  }
  n228 = disable-structure shown="Disabled" {
    disable-tunnel: w2 -> [w450 _]
    frame Disabled {
      n229 = while "Excitation laser intensity feedback measurement (all lasers)" {
        shift-right: [w451] -> _
        shift-left: w450 -> [w456]
        stop <- FALSE stop-if-true
        n230 = flat-sequence {
          tunnel: w456 -> [w458]
          tunnel: [w459] -> w454
          tunnel: [w458] -> w452
          tunnel: [w465] -> w455
          tunnel: w454 -> [w465]
          tunnel: [w464] -> w453
          tunnel: w452 -> [w464]
          tunnel: [w477] -> w451
          tunnel: w455 -> [w488]
          tunnel: w453 -> [w485]
          frame #0 {
            n231 = call "Loop Timer9"("Count(Ticks)"=w458) -> ("Tick Count(Ticks)"=w459:u16)
          }
          frame #1 {
            # "Design note:\n\nAll lasers need to be measured at the same \ntime because the AI expansion module\ncannot independently time the measurements\nwithin our requirements: their is dead time.\n\nThis probably wouldn't be an issue with the built\nin AI on the fpga board itself."
            n232 = xnode "FPGA I/O Node"("Connector1/DIO35"=TRUE) -> ("Chassis2/Mod2/AI2"=→"Blue Intensity":i16, "Chassis2/Mod2/AI1"=→"Red FB Intensity":i16, "Chassis2/Mod2/AI0"=→"Green FB Sum":i16)  [unwired: 4 in, 4 out]
          }
          frame #2 {
            n233 = feedback-in #16(w488) -> ()
            n234 = feedback #16(w488) -> (w487:u16)
            n235 = Subtract(x=w488, y=w487) -> (x-y=w486:u16)
            n236 = xnode "FPGA I/O Node"("Connector1/DIO35"=FALSE) -> ()  [unwired: 1 in, 1 out]
            n237 = Subtract(x=w486, y=w485) -> (x-y=w467:u16)
            n238 = Subtract(x="Green FB Count", y=w467) -> (x-y=w481:u16)
            n239 = Number To Boolean Array(number=w467) -> (Boolean array=w468:bool[])
            n240 = Or Array Elements(Boolean array=w468) -> (logical OR=w466:bool)
            n241 = Boolean To (0,1)(Boolean="+ phase (Green FB)") -> (0, 1=w479:i16)
            n242 = Boolean To (0,1)(Boolean=w466) -> (0, 1=w473:i16)
            n243 = Multiply(x=w479, y="Phase count adjustment (Green FB)") -> (x*y=w474:i16)
            n244 = Add(x=w481, y=w474) -> (x+y=w477:u16)
            n245 = To Unsigned Byte Integer(number=w473) -> (unsigned 8bit integer=w470:u8)
            n246 = feedback #17(i16 0) -> (w476:i16)
            n247 = Subtract(x=w476, y=w474) -> (x-y=w475:i16)
            "Green FB Relative Phase" <- w475
            n248 = feedback-in #17(w475) -> ()
            n249 = feedback #18(u8 0) -> (w471:u8)
            n250 = Add(x=w470, y=w471) -> (x+y=w469:u8)
            "Green Late Counter" <- w469
            n251 = feedback-in #18(w469) -> ()
          }
        }
      }
    }
    frame Enabled {
    }
  }
  n252 = while "RF box board direct communication loop" {
    tunnel: w2 -> [_]
    stop <- FALSE stop-if-true
    n253 = case "Whether to use direct communication method (only use one method at a time)" shown="True" "Direct RF Box \nCommunication" {
      frame False {
      }
      frame True {
        n254 = case shown="True" "Update Data" {
          frame False {
          }
          frame True {
            n255 = flat-sequence {
              frame #0 {
                n256 = First Call?() -> (First Call?: T/F=w492:bool)
                n257 = case shown="True" w492 {
                  frame False {
                  }
                  frame True {
                    # "If first time data updated, be sure to set WR high\nbefore setting data and address bits."
                    n258 = flat-sequence {
                      frame #0 {
                        n259 = xnode "FPGA I/O Node"("Connector1/DIO15"=TRUE) -> ()  [unwired: 1 in, 1 out]
                      }
                      frame #1 {
                        n260 = call "Wait"("Count(Ticks)"=u8 40 ("DO Delay 3 (Ticks)")) -> ()  [unwired: 1 out]
                      }
                    }
                  }
                }
              }
              frame #1 {
                n261 = Number To Boolean Array(number="Address") -> (Boolean array=w541:bool[])
                n262 = Number To Boolean Array(number="Data BD 1") -> (Boolean array=w542:bool[])
                n263 = Number To Boolean Array(number="Data BD 2") -> (Boolean array=w511:bool[])
                n264 = Index Array(array=w542, index=7) -> (element=w526:bool)
                n265 = Index Array(array=w542, index=6) -> (element=w525:bool)
                n266 = Index Array(array=w542, index=5) -> (element=w524:bool)
                n267 = Index Array(array=w542, index=4) -> (element=w523:bool)
                n268 = Index Array(array=w542, index=3) -> (element=w522:bool)
                n269 = Index Array(array=w542, index=2) -> (element=w521:bool)
                n270 = Index Array(array=w542, index=1) -> (element=w520:bool)
                n271 = Index Array(array=w542, index=0) -> (element=w519:bool)
                n272 = Index Array(array=w541, index=5) -> (element=w518:bool)
                n273 = Index Array(array=w541, index=4) -> (element=w517:bool)
                n274 = Index Array(array=w541, index=3) -> (element=w516:bool)
                n275 = Index Array(array=w541, index=2) -> (element=w515:bool)
                n276 = Index Array(array=w541, index=1) -> (element=w514:bool)
                n277 = Index Array(array=w541, index=0) -> (element=w513:bool)
                n278 = Index Array(array=w511, index=7) -> (element=w502:bool)
                n279 = Index Array(array=w511, index=6) -> (element=w501:bool)
                n280 = Index Array(array=w511, index=5) -> (element=w500:bool)
                n281 = Index Array(array=w511, index=4) -> (element=w499:bool)
                n282 = Index Array(array=w511, index=3) -> (element=w498:bool)
                n283 = Index Array(array=w511, index=2) -> (element=w497:bool)
                n284 = Index Array(array=w511, index=1) -> (element=w496:bool)
                n285 = Index Array(array=w511, index=0) -> (element=w495:bool)
                n286 = xnode "FPGA I/O Node"("Connector1/DIO0"=w526, "Connector1/DIO1"=w525, "Connector1/DIO2"=w524, "Connector1/DIO3"=w523, "Connector1/DIO4"=w522, "Connector1/DIO5"=w521, "Connector1/DIO6"=w520, "Connector1/DIO7"=w519, "Connector1/DIO8"=w518, "Connector1/DIO9"=w517, "Connector1/DIO10"=w516, "Connector1/DIO11"=w515, "Connector1/DIO12"=w514, "Connector1/DIO13"=w513, "Connector1/DIO20"=w502, "Connector1/DIO21"=w501, "Connector1/DIO22"=w500, "Connector1/DIO23"=w499, "Connector1/DIO24"=w498, "Connector1/DIO25"=w497, "Connector1/DIO26"=w496, "Connector1/DIO27"=w495) -> ()  [unwired: 22 in, 22 out]
              }
              frame #2 {
                # "wait and then apply write signal"
                n287 = call "Wait2"("Count(Ticks)"=u8 40 ("DO Delay 1 (Ticks)")) -> ()  [unwired: 1 out]
              }
              frame #3 {
                # "sending bit low writes data to board buffer"
                n288 = xnode "FPGA I/O Node"("Connector1/DIO15"=FALSE) -> ()  [unwired: 1 in, 1 out]
              }
              frame #4 {
                # "wait then return write signal"
                n289 = call "Wait3"("Count(Ticks)"=u8 40 ("DO Delay 2 (Ticks)")) -> ()  [unwired: 1 out]
              }
              frame #5 {
                # "sending bit high makes ready to\nwrite more data"
                n290 = xnode "FPGA I/O Node"("Connector1/DIO15"=TRUE) -> ()  [unwired: 1 in, 1 out]
              }
            }
          }
        }
      }
    }
  }
  n291 = disable-structure shown="Disabled" {
    disable-tunnel: w6 -> [w550 _]
    disable-tunnel: w2 -> [w549 _]
    frame Disabled {
      n292 = while "APD 2 Gating" {
        shift-right: [w554] -> _
        shift-left: w549 -> [w559]
        shift-right: [w553] -> _
        shift-left: w550 -> [w551]
        stop <- FALSE stop-if-true
        n293 = flat-sequence {
          tunnel: w559 -> [w562]
          tunnel: [w563] -> w557
          tunnel: [w562] -> w555
          tunnel: [w561] -> w552
          tunnel: w551 -> [w561]
          tunnel: [w566] -> w558
          tunnel: w557 -> [w566]
          tunnel: [w565] -> w556
          tunnel: w555 -> [w565]
          tunnel: w552 -> [w564]
          tunnel: [w588] -> w554
          tunnel: w558 -> [w598]
          tunnel: w556 -> [w596]
          tunnel: [w567] -> w553
          frame #0 {
            n294 = call "Loop Timer8"("Count(Ticks)"=w562) -> ("Tick Count(Ticks)"=w563:u16)
          }
          frame #1 {
            # "Signal maybe then sent through \na transistor before APD"
            n295 = xnode "FPGA I/O Node"("Connector0/DIO8"=w564, "Connector0/DIO9"=w564, "Connector0/DIO10"=w564, "Connector0/DIO11"=w564) -> ()  [unwired: 4 in, 4 out]
            "APD2 int gate" <- w564
          }
          frame #2 {
            n296 = local read "APD Gate ON Count"() -> (w581:u16)
            n297 = local read "APD Gate OFF Count"() -> (w580:u16)
            n298 = feedback #19(TRUE) -> (w593:bool)
            n299 = feedback-in #20(w598) -> ()
            n300 = feedback #20(w598) -> (w582:u16)
            n301 = Not(x=w593) -> (.not. x?=w591:bool)
            n302 = feedback-in #19(w591) -> ()
            n303 = Subtract(x=w598, y=w582) -> (x-y=w597:u16)
            n304 = Select(t=w581, s=w591, f=w580) -> (s? t:f=w595:u16)
            n305 = Subtract(x=w597, y=w596) -> (x-y=w573:u16)
            n306 = Subtract(x=w595, y=w573) -> (x-y=w587:u16)
            n307 = Number To Boolean Array(number=w573) -> (Boolean array=w572:bool[])
            n308 = Or Array Elements(Boolean array=w572) -> (logical OR=w571:bool)
            n309 = Boolean To (0,1)(Boolean="+ phase (APD 2 Gate)") -> (0, 1=w585:i16)
            n310 = Multiply(x=w585, y="Phase count adjustment (APD 2 Gate)") -> (x*y=w583:i16)
            n311 = Boolean To (0,1)(Boolean=w571) -> (0, 1=w578:i16)
            n312 = Add(x=w587, y=w583) -> (x+y=w588:u16)
            n313 = To Unsigned Byte Integer(number=w578) -> (unsigned 8bit integer=w575:u8)
            n314 = feedback #21(i16 0) -> (w590:i16)
            n315 = Subtract(x=w590, y=w583) -> (x-y=w589:i16)
            "APD 2 Gate Relative Phase" <- w589
            n316 = feedback-in #21(w589) -> ()
            n317 = feedback #22(u8 0) -> (w576:u8)
            n318 = Add(x=w575, y=w576) -> (x+y=w574:u8)
            "APD 2 Gate Late Counter" <- w574
            n319 = feedback-in #22(w574) -> ()
            n320 = local read "APD Gate Operating Mode"() -> (w579:u8)
            n321 = case shown="2" w579 {
              tunnel: [TRUE FALSE w601] -> w568
              tunnel: w593 -> [_ _ w601]
              frame 0, Default {
              }
              frame 1 {
              }
              frame 2 {
              }
            }
            n322 = local read "Invert APD Gate"() -> (w570:bool)
            n323 = Not(x=w568) -> (.not. x?=w569:bool)
            n324 = Select(t=w569, s=w570, f=w568) -> (s? t:f=w567:bool)
          }
        }
      }
    }
    frame Enabled {
    }
  }
  n325 = disable-structure shown="Disabled" {
    disable-tunnel: w2 -> [w602 _]
    frame Disabled {
      n326 = while "APD 1 Counter" {
        tunnel: w602 -> [_]
        stop <- FALSE stop-if-true
        n327 = flat-sequence {
          frame #0 {
            n328 = xnode "FPGA I/O Method Node"("FPGA I/O In"=refnum<k21> "Connector0/DIO0" ("APD 1 DO"), "Timeout"=-1) -> ()  [unwired: 2 out]
          }
          frame #1 {
            n329 = local read "APD1 int gate"() -> (w606:bool)
            n330 = case shown="True" w606 {
              frame False {
              }
              frame True {
                n331 = local read "APD1 out state"() -> (w607:bool)
                n332 = case shown="True" w607 {
                  frame False {
                    n333 = local read "APD 1 Counts 0"() -> (w609:u32)
                    n334 = Increment(x=w609) -> (x+1=→"APD 1 Counts 0":u32)
                  }
                  frame True {
                    n335 = local read "APD 1 Counts 1"() -> (w611:u32)
                    n336 = Increment(x=w611) -> (x+1=→"APD 1 Counts 1":u32)
                  }
                }
              }
            }
          }
        }
      }
      n337 = while "APD 2 Counter" {
        tunnel: w602 -> [_]
        stop <- FALSE stop-if-true
        n338 = flat-sequence {
          frame #0 {
            n339 = xnode "FPGA I/O Method Node"("FPGA I/O In"=refnum<k21> "Connector0/DIO1" ("APD 2 DO"), "Timeout"=-1) -> ()  [unwired: 2 out]
          }
          frame #1 {
            n340 = local read "APD2 int gate"() -> (w615:bool)
            n341 = case shown="True" w615 {
              frame False {
              }
              frame True {
                n342 = local read "APD2 out state"() -> (w616:bool)
                n343 = case shown="False" w616 {
                  frame False {
                    n344 = local read "APD 2 Counts 0"() -> (w618:u32)
                    n345 = Increment(x=w618) -> (x+1=→"APD 2 Counts 0":u32)
                  }
                  frame True {
                    n346 = local read "APD 2 Counts 1"() -> (w620:u32)
                    n347 = Increment(x=w620) -> (x+1=→"APD 2 Counts 1":u32)
                  }
                }
              }
            }
          }
        }
      }
    }
    frame Enabled {
    }
  }
  n348 = disable-structure shown="Disabled" {
    disable-tunnel: w6 -> [w622 _]
    disable-tunnel: w2 -> [w621 _]
    frame Disabled {
      n349 = while "APD 1 Gating" {
        shift-right: [w626] -> _
        shift-left: w621 -> [w631]
        shift-right: [w625] -> _
        shift-left: w622 -> [w623]
        stop <- FALSE stop-if-true
        n350 = flat-sequence {
          tunnel: w631 -> [w634]
          tunnel: [w635] -> w629
          tunnel: [w634] -> w627
          tunnel: [w633] -> w624
          tunnel: w623 -> [w633]
          tunnel: [w638] -> w630
          tunnel: w629 -> [w638]
          tunnel: [w637] -> w628
          tunnel: w627 -> [w637]
          tunnel: w624 -> [w636]
          tunnel: [w656] -> w626
          tunnel: w630 -> [w670]
          tunnel: w628 -> [w667]
          tunnel: [w639] -> w625
          frame #0 {
            n351 = call "Loop Timer7"("Count(Ticks)"=w634) -> ("Tick Count(Ticks)"=w635:u16)
          }
          frame #1 {
            # "Signal maybe then sent through \na transistor before APD"
            n352 = xnode "FPGA I/O Node"("Connector0/DIO4"=w636, "Connector0/DIO5"=w636, "Connector0/DIO6"=w636, "Connector0/DIO7"=w636) -> ()  [unwired: 4 in, 4 out]
            "APD1 int gate" <- w636
          }
          frame #2 {
            n353 = feedback #23(TRUE) -> (w662:bool)
            n354 = feedback-in #24(w670) -> ()
            n355 = feedback #24(w670) -> (w669:u16)
            n356 = Not(x=w662) -> (.not. x?=w659:bool)
            n357 = feedback-in #23(w659) -> ()
            n358 = Subtract(x=w670, y=w669) -> (x-y=w668:u16)
            n359 = Select(t="APD Gate ON Count", s=w659, f="APD Gate OFF Count") -> (s? t:f=w664:u16)
            n360 = Subtract(x=w668, y=w667) -> (x-y=w644:u16)
            n361 = Subtract(x=w664, y=w644) -> (x-y=w655:u16)
            n362 = Number To Boolean Array(number=w644) -> (Boolean array=w645:bool[])
            n363 = Or Array Elements(Boolean array=w645) -> (logical OR=w643:bool)
            n364 = Boolean To (0,1)(Boolean="+ phase (APD 1 Gate)") -> (0, 1=w653:i16)
            n365 = Boolean To (0,1)(Boolean=w643) -> (0, 1=w650:i16)
            n366 = Multiply(x=w653, y="Phase count adjustment (APD 1 Gate)") -> (x*y=w651:i16)
            n367 = To Unsigned Byte Integer(number=w650) -> (unsigned 8bit integer=w647:u8)
            n368 = Add(x=w655, y=w651) -> (x+y=w656:u16)
            n369 = feedback #25(i16 0) -> (w658:i16)
            n370 = Subtract(x=w658, y=w651) -> (x-y=w657:i16)
            "APD 1 Gate Relative Phase" <- w657
            n371 = feedback-in #25(w657) -> ()
            n372 = feedback #26(u8 0) -> (w648:u8)
            n373 = Add(x=w647, y=w648) -> (x+y=w646:u8)
            "APD 1 Gate Late Counter" <- w646
            n374 = feedback-in #26(w646) -> ()
            n375 = case shown="2" "APD Gate Operating Mode" {
              tunnel: [TRUE FALSE w673] -> w640
              tunnel: w662 -> [_ _ w673]
              frame 0, Default {
              }
              frame 1 {
              }
              frame 2 {
              }
            }
            n376 = Not(x=w640) -> (.not. x?=w641:bool)
            n377 = Select(t=w641, s="Invert APD Gate", f=w640) -> (s? t:f=w639:bool)
          }
        }
      }
    }
    frame Enabled {
    }
  }
  n378 = disable-structure shown="Disabled" {
    disable-tunnel: u16 0 -> [w676 _]
    disable-tunnel: w4 -> [w675 _]
    disable-tunnel: w2 -> [w674 _]
    frame Disabled {
      n379 = while "532 nm green fluorescent laser interlacing (DO to IA 532 nm AOM ME amp)." {
        shift-right: [w791] -> _
        shift-left: w674 -> [w796]
        shift-right: [w790] -> _
        shift-left: w675 -> [w788]
        stop <- FALSE stop-if-true
        n380 = flat-sequence {
          tunnel: w796 -> [w799]
          tunnel: [w800] -> w794
          tunnel: [w799] -> w792
          tunnel: [w798] -> w789
          tunnel: w788 -> [w798]
          tunnel: [w803] -> w795
          tunnel: w794 -> [w803]
          tunnel: [w802] -> w793
          tunnel: w792 -> [w802]
          tunnel: w789 -> [w801]
          tunnel: [w812] -> w791
          tunnel: w795 -> [w832]
          tunnel: w793 -> [w829]
          tunnel: [w821] -> w790
          frame #0 {
            n381 = call "Loop Timer4"("Count(Ticks)"=w799) -> ("Tick Count(Ticks)"=w800:u16)
          }
          frame #1 {
            n382 = xnode "FPGA I/O Node"("Connector1/DIO34"=w801, "Connector1/DIO38"=w801, "Connector1/DIO39"=w801) -> ()  [unwired: 3 in, 3 out]
          }
          frame #2 {
            n383 = feedback-in #27(w832) -> ()
            n384 = feedback #27(w832) -> (w831:u16)
            n385 = Subtract(x=w832, y=w831) -> (x-y=w830:u16)
            n386 = Subtract(x=w830, y=w829) -> (x-y=w805:u16)
            n387 = Number To Boolean Array(number=w805) -> (Boolean array=w806:bool[])
            n388 = Or Array Elements(Boolean array=w806) -> (logical OR=w804:bool)
            n389 = Boolean To (0,1)(Boolean="+ phase (GI)") -> (0, 1=w817:i16)
            n390 = Multiply(x=w817, y="Phase count adjustment (GI)") -> (x*y=w814:i16)
            n391 = Boolean To (0,1)(Boolean=w804) -> (0, 1=w811:i16)
            n392 = To Unsigned Byte Integer(number=w811) -> (unsigned 8bit integer=w808:u8)
            n393 = feedback #28(i16 0) -> (w815:i16)
            n394 = feedback #29(u8 0) -> (w809:u8)
            n395 = Add(x=w808, y=w809) -> (x+y=w807:u8)
            "GI Late Counter" <- w807
            n396 = feedback-in #29(w807) -> ()
            n397 = Subtract(x=w815, y=w814) -> (x-y=w813:i16)
            "GI Relative phase" <- w813
            n398 = feedback-in #28(w813) -> ()
            n399 = feedback #30(TRUE) -> (w824:bool)
            n400 = case shown="2" "Operating Mode" {
              tunnel: [TRUE FALSE w838] -> w821
              tunnel: w824 -> [_ _ w835]
              frame 0, Default {
              }
              frame 1 {
              }
              frame 2 {
                n401 = Not(x=w835) -> (.not. x?=w837:bool)
                n402 = Select(t=w837, s="Invert GI", f=w835) -> (s? t:f=w838:bool)
              }
            }
            n403 = Not(x=w824) -> (.not. x?=w820:bool)
            n404 = Select(t="Green interlace ON count", s=w820, f="Green interlace OFF count") -> (s? t:f=w826:u16)
            n405 = Subtract(x=w826, y=w805) -> (x-y=w818:u16)
            n406 = Add(x=w818, y=w814) -> (x+y=w812:u16)
            n407 = feedback-in #30(w820) -> ()
          }
        }
      }
      n408 = while "Green and red fluorescent laser interlacing (Current AO to IA 532 nm AOM ME amp)." {
        shift-right: [w685] -> _
        shift-left: w674 -> [w688]
        shift-right: [w682] -> _
        shift-left: w676 -> [w680]
        shift-right: [w679] -> _
        shift-left: w676 -> [w678]
        stop <- FALSE stop-if-true
        n409 = flat-sequence {
          tunnel: w688 -> [w692]
          tunnel: [w693] -> w687
          tunnel: [w692] -> w686
          tunnel: [w691] -> w681
          tunnel: w680 -> [w691]
          tunnel: w678 -> [w690]
          tunnel: [w690] -> w677
          tunnel: [w697] -> w684
          tunnel: w687 -> [w697]
          tunnel: [w696] -> w683
          tunnel: w686 -> [w696]
          tunnel: w681 -> [w695]
          tunnel: w677 -> [w694]
          tunnel: [w710] -> w685
          tunnel: [w726] -> w682
          tunnel: w684 -> [w737]
          tunnel: w683 -> [w734]
          tunnel: [w700] -> w679
          frame #0 {
            n410 = call "Loop Timer10"("Count(Ticks)"=w692) -> ("Tick Count(Ticks)"=w693:u16)
          }
          frame #1 {
            n411 = xnode "FPGA I/O Node"("Chassis2/Mod1/AO0"=w695, "Chassis2/Mod1/AO1"=w694) -> ()  [unwired: 2 in, 2 out]
          }
          frame #2 {
            # "Design note:\n\nThese two laser controls are in the same loop\nbecause the expansion current AI cannot separately\ntime the outputs fast enough for us.  Apparently\nit is because of communication time between the\nexpansion card and the fpga.\n\nSo the two analog control signals have the same timing\nand profile, but independent amplitudes to independently\ncontrol the intensity and feedback for each laser."
            n412 = feedback #31(TRUE) -> (w698:bool)
            n413 = Not(x=w698) -> (.not. x?=w699:bool)
            n414 = feedback-in #31(w699) -> ()
            n415 = Subtract(x="Green interlace OFF count 2", y="Green int current ON count adj") -> (x-y=w719:u16)
            n416 = disable-structure shown="Disabled" {
              disable-tunnel: [w741 _] -> w700
              disable-tunnel: w698 -> [w738 _]
              frame Disabled {
                n417 = case shown="2" "RI Operating Mode 2" {
                  tunnel: [TRUE FALSE w753] -> w739
                  tunnel: w738 -> [_ _ w750]
                  frame 0, Default {
                  }
                  frame 1 {
                  }
                  frame 2 {
                    n418 = Not(x=w750) -> (.not. x?=w752:bool)
                    n419 = Select(t=w752, s="Invert RI 2", f=w750) -> (s? t:f=w753:bool)
                  }
                }
                n420 = And(x=w739, y="Red FB On/Off") -> (x .and. y?=w747:bool)
                n421 = case shown="True" w747 {
                  tunnel: "RI Current Out" -> [w754 _]
                  tunnel: [w754 w763] -> w743
                  frame False {
                  }
                  frame True {
                    n422 = local read "Red FB Intensity"() -> (w759:i16)
                    n423 = Bundle("P4"="P4", "I4"="I4", "D4"="D4") -> (w755:cluster{"P4":i16, "I4":i16, "D4":i16})  [unwired: 1 in]
                    n424 = call "Slower PID.vi"("process variable"=w759, "reset?"="Red FB Reset", "setpoint"="Red FB Setpoint", "PID gains (x 2^8)"=w755, "output range"=cluster{"output high":i16, "output low":i16} {"output high"=32767, "output low"=-32768} ("Green FB output range")) -> ("output"=w766:i16)  [unwired: 10 out]
                    n425 = To Long Integer(number=w766) -> (32bit integer=w760:i32)
                    n426 = Add(x=w760, y=32768) -> (x+y=w762:i32)
                    n427 = To Unsigned Word Integer(number=w762) -> (unsigned 16bit integer=w763:u16)
                  }
                }
                n428 = Boolean To (0,1)(Boolean=w739) -> (0, 1=w742:i16)
                n429 = To Unsigned Word Integer(number=w742) -> (unsigned 16bit integer=w744:u16)
                n430 = Multiply(x=w744, y=w743) -> (x*y=w741:u16)
              }
              frame Enabled {
              }
            }
            n431 = feedback-in #32(w737) -> ()
            n432 = feedback #32(w737) -> (w736:u16)
            n433 = Add(x="Green int current ON count adj", y="Green interlace ON count 2") -> (x+y=w720:u16)
            n434 = Subtract(x=w737, y=w736) -> (x-y=w735:u16)
            n435 = Select(t=w720, s=w699, f=w719) -> (s? t:f=w731:u16)
            n436 = Subtract(x=w735, y=w734) -> (x-y=w703:u16)
            n437 = Subtract(x=w731, y=w703) -> (x-y=w714:u16)
            n438 = case shown="2" "Operating Mode 2" {
              tunnel: [TRUE FALSE w787] -> w701
              tunnel: w698 -> [_ _ w784]
              frame 0, Default {
              }
              frame 1 {
              }
              frame 2 {
                n439 = Not(x=w784) -> (.not. x?=w786:bool)
                n440 = Select(t=w786, s="Invert GI 2", f=w784) -> (s? t:f=w787:bool)
              }
            }
            n441 = Number To Boolean Array(number=w703) -> (Boolean array=w704:bool[])
            n442 = Boolean To (0,1)(Boolean="+ phase (GI) 2") -> (0, 1=w716:i16)
            n443 = Or Array Elements(Boolean array=w704) -> (logical OR=w702:bool)
            n444 = Boolean To (0,1)(Boolean=w702) -> (0, 1=w709:i16)
            n445 = Multiply(x=w716, y="Phase count adjustment (GI) 2") -> (x*y=w712:i16)
            n446 = To Unsigned Byte Integer(number=w709) -> (unsigned 8bit integer=w705:u8)
            n447 = Add(x=w714, y=w712) -> (x+y=w710:u16)
            n448 = feedback #33(u8 0) -> (w707:u8)
            n449 = Add(x=w705, y=w707) -> (x+y=w706:u8)
            "GI Late Counter 2" <- w706
            n450 = feedback-in #33(w706) -> ()
            n451 = feedback #34(i16 0) -> (w713:i16)
            n452 = Subtract(x=w713, y=w712) -> (x-y=w711:i16)
            "GI Relative phase 2" <- w711
            n453 = feedback-in #34(w711) -> ()
            n454 = And(x=w701, y="Green FB On/Off") -> (x .and. y?=w721:bool)
            n455 = case shown="False" w721 {
              tunnel: "Current Out" -> [w768 _]
              tunnel: [w768 w777] -> w725
              frame False {
              }
              frame True {
                n456 = local read "Green FB Sum"() -> (w773:i16)
                n457 = Bundle("P3"="P3", "I3"="I3", "D3"="D3") -> (w769:cluster{"P3":i16, "I3":i16, "D3":i16})  [unwired: 1 in]
                n458 = call "Slower PID.vi"("process variable"=w773, "reset?"="Green FB Reset", "setpoint"="Green FB Setpoint", "PID gains (x 2^8)"=w769, "output range"=cluster{"output high":i16, "output low":i16} {"output high"=32767, "output low"=-32768} ("Green FB output range")) -> ("output"=w780:i16)  [unwired: 10 out]
                n459 = To Long Integer(number=w780) -> (32bit integer=w774:i32)
                n460 = Add(x=w774, y=32768) -> (x+y=w776:i32)
                n461 = To Unsigned Word Integer(number=w776) -> (unsigned 16bit integer=w777:u16)
              }
            }
            n462 = Boolean To (0,1)(Boolean=w701) -> (0, 1=w727:i16)
            n463 = To Unsigned Word Integer(number=w727) -> (unsigned 16bit integer=w724:u16)
            n464 = Multiply(x=w724, y=w725) -> (x*y=w726:u16)
          }
        }
      }
    }
    frame Enabled {
    }
  }
  n465 = while "MCL stage control" {
    shift-right: [w862] -> _
    shift-left: w2 -> [w865]
    shift-right: [w855] -> _
    shift-left: w11 -> [w852]
    shift-right: [w854] -> _
    shift-left: w10 -> [w850]
    shift-right: [w847] -> _
    shift-left: w1 -> [w843]
    shift-right: [w846] -> _
    shift-left: w1 -> [w841]
    shift-right: [w845] -> _
    shift-left: w1 -> [w839]
    stop <- FALSE stop-if-true
    n466 = flat-sequence {
      tunnel: w865 -> [w872]
      tunnel: [w873] -> w861
      tunnel: [w872] -> w859
      tunnel: [w871] -> w853
      tunnel: w852 -> [w871]
      tunnel: [w870] -> w851
      tunnel: w850 -> [w870]
      tunnel: [w869] -> w844
      tunnel: w843 -> [w869]
      tunnel: [w868] -> w842
      tunnel: w841 -> [w868]
      tunnel: [w867] -> w840
      tunnel: w839 -> [w867]
      tunnel: w861 -> [w880]
      tunnel: [w880] -> w860
      tunnel: w859 -> [w879]
      tunnel: [w879] -> w858
      tunnel: w853 -> [w878]
      tunnel: w851 -> [w877]
      tunnel: w844 -> [w876]
      tunnel: w842 -> [w875]
      tunnel: w840 -> [w874]
      tunnel: w860 -> [w894]
      tunnel: w858 -> [w893]
      tunnel: [w894] -> w864
      tunnel: [w893] -> w863
      tunnel: [w892] -> w857
      tunnel: [w891] -> w856
      tunnel: [w885] -> w849
      tunnel: [w884] -> w848
      tunnel: [w1001] -> w862
      tunnel: w864 -> [w1008]
      tunnel: w863 -> [w1005]
      tunnel: w857 -> [w1003]
      tunnel: w856 -> [w1002]
      tunnel: [w1003] -> w855
      tunnel: [w1002] -> w854
      tunnel: w849 -> [w984]
      tunnel: w848 -> [w983]
      tunnel: ["Piezo Trap ON/Off (AO3)"] -> w847
      tunnel: [w984] -> w846
      tunnel: [w983] -> w845
      frame #0 {
        n467 = call "Loop Timer5"("Count(Ticks)"=w872) -> ("Tick Count(Ticks)"=w873:u32)
      }
      frame #1 {
        n468 = xnode "FPGA I/O Node"("Connector0/AO1"=w878, "Connector0/AO2"=w877, "Connector0/AO3"=w876, "Connector0/AO4"=w875, "Connector0/AO5"=w874) -> ()  [unwired: 5 in, 5 out]
      }
      frame #2 {
        n469 = local read "Scanning MCL"() -> (w906:bool)
        n470 = Or(x=w906, y="Start scan (MCL)") -> (x .or. y?=w901:bool)
        n471 = Not(x="Abort scan (MCL)") -> (.not. x?=w899:bool)
        n472 = And(x=w899, y=w901) -> (x .and. y?=w898:bool)
        n473 = case "Raster scan" shown="False" w898 {
          tunnel: [w939 w982] -> w903
          tunnel: "Start scan (MCL)" -> [_ w967]
          tunnel: [w939 w943] -> w887
          frame False {
            w939 = i16 0
            n474 = local write "Scanning MCL"(FALSE ("scanning")) -> ()
          }
          frame True {
            w953 = i16 0
            w952 = u64 0
            # "scan incr."
            # "freq. incr. mult."
            # "count steps"
            # "count number of cycles"
            n475 = feedback #35(w952) -> (w979:u64)
            n476 = Select(t=w952, s=w967, f=w979) -> (s? t:f=w981:u64)
            n477 = Increment(x=w981) -> (x+1=w978:u64)
            n478 = Greater?(x="Cycles per step (MCL)", y=w978) -> (0:w962:bool)
            n479 = Select(t=w978, s=w962, f=w952) -> (s? t:f=w977:u64)
            n480 = feedback-in #35(w977) -> ()
            n481 = feedback #36(w952) -> (w976:u64)
            n482 = Select(t=w952, s=w967, f=w976) -> (s? t:f=w971:u64)
            n483 = Increment(x=w971) -> (x+1=w975:u64)
            n484 = Add(x="Scan steps (MCL)", y="Scan steps (MCL)") -> (x+y=w974:u64)
            n485 = Select(t=w971, s=w962, f=w975) -> (s? t:f=w957:u64)
            n486 = Greater?(x=w974, y=w957) -> (0:w956:bool)
            n487 = Select(t=w957, s=w956, f=w952) -> (s? t:f=w972:u64)
            n488 = feedback-in #36(w972) -> ()
            n489 = Equal?(x="Scan steps (MCL)", y=w957) -> (x = y?=w961:bool)
            n490 = Greater?(x="Scan steps (MCL)", y=w971) -> (0:w970:bool)
            n491 = feedback #37(w953) -> (w973:i16)
            n492 = Select(t=w953, s=w967, f=w973) -> (s? t:f=w959:i16)
            n493 = Increment(x=w959) -> (x+1=w969:i16)
            n494 = Decrement(x=w959) -> (x-1=w968:i16)
            n495 = Select(t=w969, s=w970, f=w968) -> (s? t:f=w960:i16)
            n496 = Select(t=w959, s=w961, f=w960) -> (s? t:f=w958:i16)
            n497 = Select(t=w959, s=w962, f=w958) -> (s? t:f=w954:i16)
            n498 = Select(t=w954, s=w956, f=w953) -> (s? t:f=w955:i16)
            n499 = feedback-in #37(w955) -> ()
            n500 = feedback #38(w952) -> (w966:u64)
            n501 = Select(t=w952, s=w967, f=w966) -> (s? t:f=w941:u64)
            n502 = Increment(x=w941) -> (x+1=w963:u64)
            n503 = Select(t=w941, s=w956, f=w963) -> (s? t:f=w942:u64)
            n504 = Greater?(x="Number of scans (MCL)", y=w942) -> (0:w949:bool)
            n505 = Multiply(x="Scan freq.  increment (MCL)", y=w959) -> (x*y=w982:i16)
            n506 = Select(t=TRUE, s="Cont. Scan (MCL)", f=w949) -> (s? t:f=w948:bool)
            "Scanning MCL" <- w948
            n507 = Select(t=w942, s=w948, f=w952) -> (s? t:f=w964:u64)
            n508 = feedback-in #38(w964) -> ()
            n509 = Increment(x=w942) -> (x+1=→"Scan I (MCL)":u64)
            n510 = To Word Integer(number=w941) -> (16bit integer=w944:i16)
            n511 = Multiply(x=w944, y="Scan freq.  increment (MCL)") -> (x*y=w943:i16)
          }
        }
        n512 = case shown="True" "Multiple trap 3 position offset \nfile" {
          tunnel: ["Piezo Trap Y (AO4)" w914] -> w882
          tunnel: ["Piezo Trap X (AO5)" w912] -> w881
          frame False {
          }
          frame True {
            n513 = local read "Scan I"() -> (w911:u64)
            n514 = Decrement(x=w911) -> (x-1=w910:u64)
            n515 = Quotient & Remainder(x=w910, y="Piezo offset Y points") -> (x-y*floor(x/y)=w921:u64, floor(x/y)=w922:u64)
            n516 = Multiply(x=w921, y="Piezo Offset Increment") -> (x*y=w919:u64)
            n517 = Multiply(x="Piezo Offset Increment", y=w922) -> (x*y=w920:u64)
            n518 = Add(x=w920, y="Piezo offset Xmin") -> (x+y=w913:u64)
            n519 = Add(x=w919, y="Piezo Offset Ymin") -> (x+y=w915:u64)
            n520 = To Word Integer(number=w915) -> (16bit integer=w914:i16)
            n521 = To Word Integer(number=w913) -> (16bit integer=w912:i16)
          }
        }
        n522 = Select(t=w887, s="1D or 2D Scan?", f=i16 0) -> (s? t:f=w888:i16)
        n523 = Select(t=w903, s="MCL Scan Axis", f=w888) -> (s? t:f=w904:i16)
        n524 = Select(t=w888, s="MCL Scan Axis", f=w903) -> (s? t:f=w902:i16)
        n525 = case shown="False" "ScanTrap 3 or Fl-laser" {
          tunnel: w904 -> [w930 w932]
          tunnel: w902 -> [w929 w936]
          tunnel: "AO2 (X)" -> [w928 w937]
          tunnel: "AO1 (Y)" -> [w927 w938]
          tunnel: [w926 w938] -> w892
          tunnel: [w925 w937] -> w891
          tunnel: w882 -> [w924 w933]
          tunnel: [w924 w931] -> w885
          tunnel: w881 -> [w923 w935]
          tunnel: [w923 w934] -> w884
          frame False {
            n526 = Add(x=w927, y=w930) -> (x+y=w926:i16)
            n527 = Add(x=w929, y=w928) -> (x+y=w925:i16)
          }
          frame True {
            n528 = Add(x=w933, y=w932) -> (x+y=w931:i16)
            n529 = Add(x=w935, y=w936) -> (x+y=w934:i16)
          }
        }
      }
      frame #3 {
        n530 = feedback-in #39(w1008) -> ()
        n531 = feedback #39(w1008) -> (w1007:u32)
        n532 = Boolean To (0,1)(Boolean="+ phase (MCL)") -> (0, 1=w999:i16)
        n533 = Subtract(x=w1008, y=w1007) -> (x-y=w1006:u32)
        n534 = Multiply(x=w999, y="Phase count adjustment (MCL)") -> (x*y=w995:i16)
        n535 = Subtract(x=w1006, y=w1005) -> (x-y=w987:u32)
        n536 = Subtract(x="MCL count", y=w987) -> (x-y=w997:u32)
        n537 = feedback #40(i16 0) -> (w996:i16)
        n538 = Subtract(x=w996, y=w995) -> (x-y=w994:i16)
        "MCL Relative Phase" <- w994
        n539 = feedback-in #40(w994) -> ()
        n540 = Number To Boolean Array(number=w987) -> (Boolean array=w988:bool[])
        n541 = Or Array Elements(Boolean array=w988) -> (logical OR=w986:bool)
        n542 = Boolean To (0,1)(Boolean=w986) -> (0, 1=w993:i16)
        n543 = Add(x=w997, y=w995) -> (x+y=w1001:u32)
        n544 = To Unsigned Byte Integer(number=w993) -> (unsigned 8bit integer=w990:u8)
        n545 = feedback #41(u8 0) -> (w991:u8)
        n546 = Add(x=w990, y=w991) -> (x+y=w989:u8)
        "MCL Late Counter" <- w989
        n547 = feedback-in #41(w989) -> ()
        "Piezo Y out" <- w984
        "Piezo X out" <- w983
      }
    }
  }
  n548 = while "Control APD data integration - stream to host" {
    shift-right: [w1013] -> _
    shift-left: w7 -> [w1018]
    stop <- FALSE stop-if-true
    n549 = flat-sequence {
      tunnel: w1018 -> [w1020]
      tunnel: [w1021] -> w1016
      tunnel: [w1020] -> w1014
      tunnel: [w1031] -> w1017
      tunnel: w1016 -> [w1031]
      tunnel: [w1030] -> w1015
      tunnel: w1014 -> [w1030]
      tunnel: [w1029] -> w1012
      tunnel: [w1028] -> w1011
      tunnel: [w1022] -> w1010
      tunnel: [w1073] -> w1013
      tunnel: w1017 -> [w1083]
      tunnel: w1015 -> [w1080]
      tunnel: w1012 -> [w1066]
      tunnel: w1011 -> [w1065]
      tunnel: w1010 -> [w1053]
      frame #0 {
        n550 = call "Loop Timer6"("Count(Ticks)"=w1020) -> ("Tick Count(Ticks)"=w1021:u32)
      }
      frame #1 {
        n551 = flat-sequence {
          tunnel: [w1033] -> w1027
          tunnel: w1027 -> [w1036]
          tunnel: [w1040] -> w1026
          tunnel: [w1039] -> w1025
          tunnel: [w1036] -> w1024
          tunnel: [w1035] -> w1023
          tunnel: [w1047] -> w1028
          tunnel: [w1048] -> w1029
          tunnel: w1026 -> [w1048]
          tunnel: w1025 -> [w1047]
          tunnel: w1024 -> [w1046]
          tunnel: w1023 -> [w1045]
          tunnel: [w1045] -> w1022
          frame #0 {
            # "use separate variable so each APD won't\nhave to wait to read"
            n552 = feedback #42(FALSE) -> (w1032:bool)
            "APD1 out state" <- w1032
            "APD2 out state" <- w1032
            "APD3 out state" <- w1032
            n553 = Not(x=w1032) -> (.not. x?=w1033:bool)
            n554 = feedback-in #42(w1033) -> ()
          }
          frame #1 {
            n555 = local read "APD 3 Counts 1"() -> (w1038:u32)
            n556 = local read "APD 3 Counts 0"() -> (w1037:u32)
            n557 = local read "APD 1 Counts 1"() -> (w1044:u32)
            n558 = local read "APD 1 Counts 0"() -> (w1043:u32)
            n559 = local read "APD 2 Counts 1"() -> (w1042:u32)
            n560 = local read "APD 2 Counts 0"() -> (w1041:u32)
            n561 = Select(t=w1038, s=w1036, f=w1037) -> (s? t:f=w1035:u32)
            n562 = Select(t=w1044, s=w1036, f=w1043) -> (s? t:f=w1040:u32)
            n563 = Select(t=w1042, s=w1036, f=w1041) -> (s? t:f=w1039:u32)
          }
          frame #2 {
            n564 = case shown="False" w1046 {
              frame False {
                w1049 = u32 0 ("APD 1 Counts 0")
                n565 = local write "APD 1 Counts 0"(w1049) -> ()
                n566 = local write "APD 2 Counts 0"(w1049) -> ()
                n567 = local write "APD 3 Counts 0"(w1049) -> ()
              }
              frame True {
                w1050 = u32 0 ("APD 1 Counts 1")
                n568 = local write "APD 1 Counts 1"(w1050) -> ()
                n569 = local write "APD 2 Counts 1"(w1050) -> ()
                n570 = local write "APD 3 Counts 1"(w1050) -> ()
              }
            }
          }
        }
      }
      frame #2 {
        n571 = feedback-in #43(w1083) -> ()
        n572 = feedback #43(w1083) -> (w1082:u32)
        n573 = Subtract(x=w1083, y=w1082) -> (x-y=w1081:u32)
        n574 = Subtract(x=w1081, y=w1080) -> (x-y=w1058:u32)
        n575 = case shown="True" "APD to FIFO" {
          tunnel: w1066 -> [_ w1088]
          tunnel: w1065 -> [_ w1086]
          tunnel: w1053 -> [_ w1084]
          frame False {
          }
          frame True {
            n576 = flat-sequence {
              tunnel: 0 ("Timeout") -> [w1090]
              tunnel: w1088 -> [w1091]
              tunnel: [w1090] -> w1087
              tunnel: w1087 -> [w1092]
              tunnel: w1086 -> [w1093]
              tunnel: [w1092] -> w1085
              tunnel: w1085 -> [w1095]
              tunnel: w1084 -> [w1094]
              frame #0 {
                n577 = xnode ("FIFO Write")("Element"=w1091, "Timeout"=w1090) -> ()  [unwired: 1 in, 2 out]
              }
              frame #1 {
                n578 = xnode ("FIFO Write")("Element"=w1093, "Timeout"=w1092) -> ()  [unwired: 1 in, 2 out]
              }
              frame #2 {
                n579 = xnode ("FIFO Write")("Element"=w1094, "Timeout"=w1095) -> ()  [unwired: 1 in, 2 out]
              }
            }
          }
        }
        n580 = Subtract(x="APD Acq Rate Count", y=w1058) -> (x-y=w1074:u32)
        n581 = Number To Boolean Array(number=w1058) -> (Boolean array=w1059:bool[])
        n582 = Or Array Elements(Boolean array=w1059) -> (logical OR=w1057:bool)
        n583 = Boolean To (0,1)(Boolean=w1057) -> (0, 1=w1064:i16)
        n584 = To Unsigned Byte Integer(number=w1064) -> (unsigned 8bit integer=w1061:u8)
        n585 = feedback #44(u8 0) -> (w1062:u8)
        n586 = Add(x=w1061, y=w1062) -> (x+y=w1060:u8)
        "APD Acq Late Counter" <- w1060
        n587 = feedback-in #44(w1060) -> ()
        n588 = Boolean To (0,1)(Boolean="+ phase (APD Acq)") -> (0, 1=w1070:i16)
        n589 = Multiply(x=w1070, y="Phase Count Adjustment (APD Acq)") -> (x*y=w1067:i16)
        n590 = Add(x=w1074, y=w1067) -> (x+y=w1073:u32)
        n591 = feedback #45(i16 0) -> (w1072:i16)
        n592 = Subtract(x=w1072, y=w1067) -> (x-y=w1069:i16)
        "APD Acq Relative Phase" <- w1069
        n593 = feedback-in #45(w1069) -> ()
        n594 = To Word Integer(number=w1066) -> (16bit integer=w1075:i16)
        n595 = To Word Integer(number=w1053) -> (16bit integer=w1054:i16)
        n596 = To Word Integer(number=w1065) -> (16bit integer=w1076:i16)
        n597 = Multiply(x="APD AO scale factor", y=w1076) -> (x*y=w1055:i16)
        n598 = Multiply(x="APD AO scale factor", y=w1054) -> (x*y=w1051:i16)
        n599 = Multiply(x="APD AO scale factor", y=w1075) -> (x*y=w1056:i16)
        n600 = xnode "FPGA I/O Node"("Connector0/AO6"=w1056, "Connector0/AO7"=w1055, "Connector0/AO5"=w1051) -> ()  [unwired: 3 in, 3 out]
      }
    }
  }
  n601 = while "DAQ AI set 1" {
    shift-right: [w1096] -> _
    shift-left: w2 -> [w1101]
    stop <- FALSE stop-if-true
    n602 = flat-sequence {
      tunnel: w1101 -> [w1111]
      tunnel: [w1112] -> w1099
      tunnel: [w1111] -> w1098
      tunnel: [w1122] -> w1109
      tunnel: [w1121] -> w1108
      tunnel: [w1120] -> w1107
      tunnel: [w1119] -> w1106
      tunnel: [w1118] -> w1105
      tunnel: [w1117] -> w1104
      tunnel: [w1116] -> w1103
      tunnel: [w1115] -> w1102
      tunnel: [w1114] -> w1100
      tunnel: w1099 -> [w1114]
      tunnel: w1098 -> [w1113]
      tunnel: [w1113] -> w1097
      tunnel: [w1154] -> w1096
      tunnel: w1109 -> [w1180]
      tunnel: w1108 -> [w1146]
      tunnel: w1107 -> [w1147]
      tunnel: w1106 -> [w1127]
      tunnel: w1105 -> [w1170]
      tunnel: w1104 -> [w1169]
      tunnel: w1103 -> [w1168]
      tunnel: w1102 -> [w1167]
      tunnel: w1100 -> [w1164]
      tunnel: w1097 -> [w1161]
      frame #0 {
        n603 = call "Loop Timer3"("Count(Ticks)"=w1111) -> ("Tick Count(Ticks)"=w1112:u16)
      }
      frame #1 {
        n604 = xnode "FPGA I/O Node"("Connector1/DIO31"=TRUE ("Connector1/DIO33")) -> ("Connector0/AI0"=w1122:i16, "Connector0/AI1"=w1121:i16, "Connector0/AI2"=w1120:i16, "Connector0/AI3"=w1119:i16, "Connector0/AI4"=w1118:i16, "Connector0/AI5"=w1117:i16, "Connector0/AI6"=w1116:i16, "Connector0/AI7"=w1115:i16)  [unwired: 9 in, 9 out]
      }
      frame #2 {
        w1150 = FALSE ("AI to FIFO")
        # "Changed by Ronen - the X and Y values of the MCL trap are now sent to the trap position FIFO"
        # "Adjust phase after data acquired if button pressed"
        n605 = feedback #46(i16 1) -> (w1173:i16)
        n606 = Increment(x=w1173) -> (x+1=w1179:i16)
        n607 = Scale By Power Of 2(n="AI1 X Scale", x=w1146) -> (x*2^n=w1144:i16)
        n608 = Greater?(x=w1179, y="N of AI1 Int Acq Sets") -> (0:w1176:bool)
        n609 = Select(t=i16 1, s=w1176, f=w1179) -> (s? t:f=w1178:i16)
        n610 = feedback-in #46(w1178) -> ()
        n611 = Divide(x=w1144, y=w1127) -> (x/y=w1143:fxp<+/-,16,1>)
        n612 = feedback #47(w1150) -> (w1148:bool)
        n613 = feedback #48(w1150) -> (w1166:bool)
        n614 = case shown="1, Default" w1173 {
          tunnel: w1147 -> [w1205 w1212 _]
          tunnel: ["Set 1" "Set 2" "Set 3"] -> w1171
          tunnel: ["AI to FIFO" w1214 w1219] -> w1165
          tunnel: w1166 -> [_ w1214 w1219]
          tunnel: ["Trap Pos to FIFO" w1213 w1218] -> w1149
          tunnel: w1148 -> [_ w1213 w1218]
          tunnel: w1143 -> [w1204 w1211 _]
          tunnel: [w1203 w1209 FALSE] -> w1126
          tunnel: [w1202 w1210 u64 0 ("BD1 Frequency Out 2")] -> w1130
          frame 1, Default {
            n615 = local read "BD1 Frequency Out 1"() -> (w1202:u64)
            n616 = Compound Arithmetic op=AND("Trap Pos to FIFO", "Set 1", "AI to FIFO") -> (w1203:bool)
            "AI2 Y Sum Set 1" <- w1205
            "AI1 X Set 1" <- w1204
          }
          frame 2 {
            n617 = local read "BD1 Frequency Out 2"() -> (w1210:u64)
            n618 = Compound Arithmetic op=AND(w1213, "Set 2", w1214) -> (w1209:bool)
            "AI2 Y Sum Set 2" <- w1212
            "AI1 X Set 2" <- w1211
          }
          frame 3 {
          }
        }
        n619 = And(x=w1171, y=w1165) -> (x .and. y?=w1172:bool)
        n620 = case shown="True" w1172 {
          tunnel: w1180 -> [_ w1233]
          tunnel: w1146 -> [_ w1232]
          tunnel: w1147 -> [_ w1231]
          tunnel: w1127 -> [_ w1230]
          tunnel: w1170 -> [_ w1229]
          tunnel: w1169 -> [_ w1228]
          tunnel: w1168 -> [_ w1227]
          tunnel: w1167 -> [_ w1226]
          tunnel: 0 ("DMA buffer timeout") -> [_ w1235]
          frame False {
          }
          frame True {
            n621 = Build Array(w1233, w1232, w1231, w1230, w1229, w1228, w1227, w1226) -> (w1234:i16[])
            n622 = for {
              tunnel: w1234 -> [w1237] mode=indexing
              tunnel: w1235 -> [w1238]
              tunnel: [w1236] -> w1224 mode=indexing
              n623 = xnode ("FIFO Write")("Element"=w1237, "Timeout"=w1238) -> ("Timed Out?"=w1236:bool)  [unwired: 1 in, 1 out]
            }
            n624 = Or Array Elements(Boolean array=w1224) -> (logical OR=w1221:bool)
            n625 = Boolean To (0,1)(Boolean=w1221) -> (0, 1=w1223:i16)
            n626 = feedback #49(u16 0) -> (w1222:u16)
            n627 = Add(x=w1223, y=w1222) -> (x+y=w1220:u16)
            "Trap AI FIFO Timeout" <- w1220
            n628 = feedback-in #49(w1220) -> ()
          }
        }
        n629 = feedback-in #47(w1149) -> ()
        n630 = feedback-in #48(w1165) -> ()
        n631 = local read "Piezo Y out"() -> (w1124:i16)
        n632 = local read "Piezo X out"() -> (w1125:i16)
        n633 = case shown="True" w1126 {
          tunnel: w1130 -> [_ w1188]
          tunnel: [u8 0 w1185] -> w1129
          tunnel: w1125 -> [_ w1184]
          tunnel: w1124 -> [_ w1183]
          frame False {
          }
          frame True {
            n634 = Split Number(x=w1188) -> (hi(x)=w1189:u32, lo(x)=w1190:u32)
            n635 = Split Number(x=w1189) -> (lo(x)=w1191:u16)  [unwired: 1 out]
            n636 = Split Number(x=w1190) -> (hi(x)=w1192:u16, lo(x)=w1193:u16)
            n637 = Build Array "BD 1 nu Stack"(w1191, w1192, w1193, w1184, w1183) -> (w1187:u16[])
            n638 = for {
              tunnel: w1187 -> [w1200] mode=indexing
              shift-right: [w1196] -> w1185
              shift-left: u8 0 -> [w1197]
              n639 = xnode ("FIFO Method Node")("Element"=w1200, "Timeout"="Trap FIFO Set Timeout") -> ("Timed Out?"=w1199:bool)  [unwired: 1 in, 1 out]
              n640 = Boolean To (0,1)(Boolean=w1199) -> (0, 1=w1198:i16)
              n641 = To Unsigned Byte Integer(number=w1198) -> (unsigned 8bit integer=w1195:u8)
              n642 = Add(x=w1195, y=w1197) -> (x+y=w1196:u8)
            }
          }
        }
        n643 = To Unsigned Word Integer(number=w1129) -> (unsigned 16bit integer=w1128:u16)
        n644 = feedback #50(u16 0) -> (w1141:u16)
        n645 = Add(x=w1128, y=w1141) -> (x+y=w1140:u16)
        "Trap Pos FIFO Timeout" <- w1140
        n646 = feedback-in #50(w1140) -> ()
        n647 = feedback-in #51(w1164) -> ()
        n648 = feedback #51(w1164) -> (w1163:u16)
        n649 = Subtract(x=w1164, y=w1163) -> (x-y=w1162:u16)
        n650 = xnode "FPGA I/O Node"("Connector1/DIO31"=FALSE ("Connector1/DIO34")) -> ()  [unwired: 1 in, 1 out]
        n651 = Subtract(x=w1162, y=w1161) -> (x-y=w1132:u16)
        n652 = Boolean To (0,1)(Boolean="+ phase") -> (0, 1=w1157:i16)
        n653 = Multiply(x=w1157, y="Phase count adjustment") -> (x*y=w1151:i16)
        n654 = Subtract(x="ai count", y=w1132) -> (x-y=w1155:u16)
        n655 = Number To Boolean Array(number=w1132) -> (Boolean array=w1133:bool[])
        n656 = feedback #52(i16 0) -> (w1153:i16)
        n657 = Add(x=w1155, y=w1151) -> (x+y=w1154:u16)
        n658 = Subtract(x=w1153, y=w1151) -> (x-y=w1152:i16)
        "Relative phase" <- w1152
        n659 = feedback-in #52(w1152) -> ()
        n660 = Or Array Elements(Boolean array=w1133) -> (logical OR=w1131:bool)
        n661 = Boolean To (0,1)(Boolean=w1131) -> (0, 1=w1138:i16)
        n662 = To Unsigned Byte Integer(number=w1138) -> (unsigned 8bit integer=w1135:u8)
        n663 = feedback #53(u8 0) -> (w1136:u8)
        n664 = Add(x=w1135, y=w1136) -> (x+y=w1134:u8)
        "AI Late Counter" <- w1134
        n665 = feedback-in #53(w1134) -> ()
      }
    }
  }
  n666 = node-c288(w8) -> ()
  n667 = disable-structure shown="Disabled" {
    disable-tunnel: w2 -> [w1239 _]
    frame Disabled {
      n668 = while "APD 3 Counter" {
        tunnel: w1239 -> [_]
        stop <- FALSE stop-if-true
        n669 = flat-sequence {
          frame #0 {
            n670 = xnode "FPGA I/O Method Node"("FPGA I/O In"=refnum<k21> "Connector0/DIO2" ("APD 2 DO"), "Timeout"=-1) -> ()  [unwired: 2 out]
          }
          frame #1 {
            n671 = local read "APD3 int gate"() -> (w1243:bool)
            n672 = case shown="True" w1243 {
              frame False {
              }
              frame True {
                n673 = local read "APD3 out state"() -> (w1244:bool)
                n674 = case shown="True" w1244 {
                  frame False {
                    n675 = local read "APD 3 Counts 0"() -> (w1246:u32)
                    n676 = Increment(x=w1246) -> (x+1=→"APD 3 Counts 0":u32)
                  }
                  frame True {
                    n677 = local read "APD 3 Counts 1"() -> (w1248:u32)
                    n678 = Increment(x=w1248) -> (x+1=→"APD 3 Counts 1":u32)
                  }
                }
              }
            }
          }
        }
      }
    }
    frame Enabled {
    }
  }
  n679 = disable-structure shown="Disabled" {
    disable-tunnel: w6 -> [w1250 _]
    disable-tunnel: w2 -> [w1249 _]
    frame Disabled {
      n680 = while "APD 3 Gating" {
        shift-right: [w1254] -> _
        shift-left: w1249 -> [w1259]
        shift-right: [w1253] -> _
        shift-left: w1250 -> [w1251]
        stop <- FALSE stop-if-true
        n681 = flat-sequence {
          tunnel: w1259 -> [w1262]
          tunnel: [w1263] -> w1257
          tunnel: [w1262] -> w1255
          tunnel: [w1261] -> w1252
          tunnel: w1251 -> [w1261]
          tunnel: [w1266] -> w1258
          tunnel: w1257 -> [w1266]
          tunnel: [w1265] -> w1256
          tunnel: w1255 -> [w1265]
          tunnel: w1252 -> [w1264]
          tunnel: [w1287] -> w1254
          tunnel: w1258 -> [w1298]
          tunnel: w1256 -> [w1295]
          tunnel: [w1267] -> w1253
          frame #0 {
            n682 = call "Loop Timer15"("Count(Ticks)"=w1262) -> ("Tick Count(Ticks)"=w1263:u16)
          }
          frame #1 {
            # "Signal maybe then sent through \na transistor before APD"
            n683 = xnode "FPGA I/O Node"("Connector0/DIO12"=w1264, "Connector0/DIO13"=w1264, "Connector0/DIO14"=w1264, "Connector0/DIO15"=w1264) -> ()  [unwired: 4 in, 4 out]
            "APD3 int gate" <- w1264
          }
          frame #2 {
            n684 = local read "APD Gate OFF Count"() -> (w1272:u16)
            n685 = local read "APD Gate ON Count"() -> (w1273:u16)
            n686 = feedback #54(TRUE) -> (w1292:bool)
            n687 = feedback-in #55(w1298) -> ()
            n688 = feedback #55(w1298) -> (w1297:u16)
            n689 = Not(x=w1292) -> (.not. x?=w1290:bool)
            n690 = feedback-in #54(w1290) -> ()
            n691 = Subtract(x=w1298, y=w1297) -> (x-y=w1296:u16)
            n692 = Select(t=w1273, s=w1290, f=w1272) -> (s? t:f=w1294:u16)
            n693 = Subtract(x=w1296, y=w1295) -> (x-y=w1275:u16)
            n694 = Subtract(x=w1294, y=w1275) -> (x-y=w1286:u16)
            n695 = Number To Boolean Array(number=w1275) -> (Boolean array=w1276:bool[])
            n696 = Or Array Elements(Boolean array=w1276) -> (logical OR=w1274:bool)
            n697 = Boolean To (0,1)(Boolean=w1274) -> (0, 1=w1281:i16)
            n698 = Boolean To (0,1)(Boolean="+ phase (APD 3 Gate)") -> (0, 1=w1284:i16)
            n699 = To Unsigned Byte Integer(number=w1281) -> (unsigned 8bit integer=w1278:u8)
            n700 = Multiply(x=w1284, y="Phase count adjustment (APD 3 Gate)") -> (x*y=w1282:i16)
            n701 = feedback #56(u8 0) -> (w1279:u8)
            n702 = Add(x=w1278, y=w1279) -> (x+y=w1277:u8)
            "APD 3 Gate Late Counter" <- w1277
            n703 = feedback-in #56(w1277) -> ()
            n704 = Add(x=w1286, y=w1282) -> (x+y=w1287:u16)
            n705 = feedback #57(i16 0) -> (w1289:i16)
            n706 = Subtract(x=w1289, y=w1282) -> (x-y=w1288:i16)
            "APD 3 Gate Relative Phase" <- w1288
            n707 = feedback-in #57(w1288) -> ()
            n708 = local read "APD Gate Operating Mode"() -> (w1271:u8)
            n709 = case shown="2" w1271 {
              tunnel: [TRUE FALSE w1301] -> w1268
              tunnel: w1292 -> [_ _ w1301]
              frame 0, Default {
              }
              frame 1 {
              }
              frame 2 {
              }
            }
            n710 = local read "Invert APD Gate"() -> (w1270:bool)
            n711 = Not(x=w1268) -> (.not. x?=w1269:bool)
            n712 = Select(t=w1269, s=w1270, f=w1268) -> (s? t:f=w1267:bool)
          }
        }
      }
    }
    frame Enabled {
    }
  }
  n713 = disable-structure shown="Disabled" {
    disable-tunnel: w4 -> [w1303 _]
    disable-tunnel: w2 -> [w1302 _]
    frame Disabled {
      n714 = while "633 nm red  fluorescent laser interlacing (DO to IA 633 nm AOM ME amp)." {
        shift-right: [w1307] -> _
        shift-left: w1302 -> [w1312]
        shift-right: [w1306] -> _
        shift-left: w1303 -> [w1304]
        stop <- FALSE stop-if-true
        n715 = flat-sequence {
          tunnel: w1312 -> [w1315]
          tunnel: [w1316] -> w1310
          tunnel: [w1315] -> w1308
          tunnel: [w1314] -> w1305
          tunnel: w1304 -> [w1314]
          tunnel: [w1319] -> w1311
          tunnel: w1310 -> [w1319]
          tunnel: [w1318] -> w1309
          tunnel: w1308 -> [w1318]
          tunnel: w1305 -> [w1317]
          tunnel: [w1328] -> w1307
          tunnel: w1311 -> [w1348]
          tunnel: w1309 -> [w1345]
          tunnel: [w1337] -> w1306
          frame #0 {
            n716 = call "Loop Timer11"("Count(Ticks)"=w1315) -> ("Tick Count(Ticks)"=w1316:u16)
          }
          frame #1 {
            # "Then to PRL 440 amp"
            n717 = xnode "FPGA I/O Node"("Connector1/DIO32"=w1317) -> ()  [unwired: 1 in, 1 out]
          }
          frame #2 {
            n718 = feedback-in #58(w1348) -> ()
            n719 = feedback #58(w1348) -> (w1347:u16)
            n720 = Subtract(x=w1348, y=w1347) -> (x-y=w1346:u16)
            n721 = Subtract(x=w1346, y=w1345) -> (x-y=w1321:u16)
            n722 = Number To Boolean Array(number=w1321) -> (Boolean array=w1322:bool[])
            n723 = Or Array Elements(Boolean array=w1322) -> (logical OR=w1320:bool)
            n724 = Boolean To (0,1)(Boolean="+ phase (RI)") -> (0, 1=w1333:i16)
            n725 = Multiply(x=w1333, y="Phase count adjustment (RI)") -> (x*y=w1330:i16)
            n726 = Boolean To (0,1)(Boolean=w1320) -> (0, 1=w1327:i16)
            n727 = To Unsigned Byte Integer(number=w1327) -> (unsigned 8bit integer=w1324:u8)
            n728 = feedback #59(i16 0) -> (w1331:i16)
            n729 = feedback #60(u8 0) -> (w1325:u8)
            n730 = Add(x=w1324, y=w1325) -> (x+y=w1323:u8)
            "RI Late Counter" <- w1323
            n731 = feedback-in #60(w1323) -> ()
            n732 = Subtract(x=w1331, y=w1330) -> (x-y=w1329:i16)
            "RI Relative phase" <- w1329
            n733 = feedback-in #59(w1329) -> ()
            n734 = feedback #61(TRUE) -> (w1340:bool)
            n735 = case shown="2" "Red Laser Operating Mode" {
              tunnel: [TRUE FALSE w1354] -> w1337
              tunnel: w1340 -> [_ _ w1351]
              frame 0, Default {
              }
              frame 1 {
              }
              frame 2 {
                n736 = Not(x=w1351) -> (.not. x?=w1353:bool)
                n737 = Select(t=w1353, s="Invert RI", f=w1351) -> (s? t:f=w1354:bool)
              }
            }
            n738 = Not(x=w1340) -> (.not. x?=w1336:bool)
            n739 = Select(t="Red interlace ON count", s=w1336, f="Red interlace OFF count") -> (s? t:f=w1342:u16)
            n740 = Subtract(x=w1342, y=w1321) -> (x-y=w1334:u16)
            n741 = Add(x=w1334, y=w1330) -> (x+y=w1328:u16)
            n742 = feedback-in #61(w1336) -> ()
          }
        }
      }
    }
    frame Enabled {
    }
  }
  n743 = disable-structure shown="Disabled" {
    disable-tunnel: w2 -> [w1355 _]
    frame Disabled {
      n744 = while "Blue fluorescent laser interlacing (AO control direct to laser)." {
        shift-right: [w1362] -> _
        shift-left: w1355 -> [w1365]
        shift-right: [w1359] -> _
        shift-left: i16 0 -> [w1357]
        stop <- FALSE stop-if-true
        n745 = flat-sequence {
          tunnel: w1365 -> [w1368]
          tunnel: [w1369] -> w1364
          tunnel: [w1368] -> w1363
          tunnel: [w1367] -> w1358
          tunnel: w1357 -> [w1367]
          tunnel: [w1372] -> w1361
          tunnel: w1364 -> [w1372]
          tunnel: [w1371] -> w1360
          tunnel: w1363 -> [w1371]
          tunnel: w1358 -> [w1370]
          tunnel: [w1382] -> w1362
          tunnel: [w1398] -> w1359
          tunnel: w1361 -> [w1410]
          tunnel: w1360 -> [w1407]
          frame #0 {
            n746 = call "Loop Timer13"("Count(Ticks)"=w1368) -> ("Tick Count(Ticks)"=w1369:u16)
          }
          frame #1 {
            n747 = xnode "FPGA I/O Node"("Connector0/AO3"=w1370) -> ()  [unwired: 1 in, 1 out]
          }
          frame #2 {
            n748 = Subtract(x="Blue OFF count (AO)", y="Blue current ON count adj (AO)") -> (x-y=w1391:u16)
            n749 = feedback-in #62(w1410) -> ()
            n750 = feedback #62(w1410) -> (w1409:u16)
            n751 = Add(x="Blue current ON count adj (AO)", y="Blue ON count (AO)") -> (x+y=w1392:u16)
            n752 = Subtract(x=w1410, y=w1409) -> (x-y=w1408:u16)
            n753 = Subtract(x=w1408, y=w1407) -> (x-y=w1375:u16)
            n754 = Number To Boolean Array(number=w1375) -> (Boolean array=w1376:bool[])
            n755 = Boolean To (0,1)(Boolean="+ phase (BI AO)") -> (0, 1=w1388:i16)
            n756 = Or Array Elements(Boolean array=w1376) -> (logical OR=w1374:bool)
            n757 = Boolean To (0,1)(Boolean=w1374) -> (0, 1=w1381:i16)
            n758 = Multiply(x=w1388, y="Phase count adjustment (BI AO)") -> (x*y=w1384:i16)
            n759 = To Unsigned Byte Integer(number=w1381) -> (unsigned 8bit integer=w1377:u8)
            n760 = feedback #63(u8 0) -> (w1379:u8)
            n761 = Add(x=w1377, y=w1379) -> (x+y=w1378:u8)
            "BI Late Counter (AO)" <- w1378
            n762 = feedback-in #63(w1378) -> ()
            n763 = feedback #64(i16 0) -> (w1385:i16)
            n764 = Subtract(x=w1385, y=w1384) -> (x-y=w1383:i16)
            "BI Relative phase (AO)" <- w1383
            n765 = feedback-in #64(w1383) -> ()
            n766 = feedback #65(TRUE) -> (w1402:bool)
            n767 = case shown="2" "BI Operating Mode (AO)" {
              tunnel: [TRUE FALSE w1426] -> w1393
              tunnel: w1402 -> [_ _ w1423]
              frame 0, Default {
              }
              frame 1 {
              }
              frame 2 {
                n768 = Not(x=w1423) -> (.not. x?=w1425:bool)
                n769 = Select(t=w1425, s="Invert BI (AO)", f=w1423) -> (s? t:f=w1426:bool)
              }
            }
            n770 = And(x=w1393, y="Blue FB On/Off") -> (x .and. y?=w1394:bool)
            n771 = case shown="True" w1394 {
              tunnel: "BI Current Out" -> [w1411 _]
              tunnel: [w1411 w1413] -> w1397
              frame False {
              }
              frame True {
                n772 = local read "Blue Intensity"() -> (w1412:i16)
                n773 = Bundle("P5"="P5", "I5"="I5", "D5"="D5") -> (w1414:cluster{"P5":i16, "I5":i16, "D5":i16})  [unwired: 1 in]
                n774 = call "Slower PID.vi"("process variable"=w1412, "reset?"="Blue FB Reset", "setpoint"="Blue FB Setpoint", "PID gains (x 2^8)"=w1414, "output range"=cluster{"output high":i16, "output low":i16} {"output high"=32767, "output low"=0} ("Green FB output range")) -> ("output"=w1413:i16)  [unwired: 10 out]
              }
            }
            n775 = Not(x=w1402) -> (.not. x?=w1399:bool)
            n776 = Select(t=w1392, s=w1399, f=w1391) -> (s? t:f=w1404:u16)
            n777 = Subtract(x=w1404, y=w1375) -> (x-y=w1386:u16)
            n778 = Add(x=w1386, y=w1384) -> (x+y=w1382:u16)
            n779 = feedback-in #65(w1399) -> ()
            n780 = Boolean To (0,1)(Boolean=w1393) -> (0, 1=w1373:i16)
            n781 = Multiply(x=w1373, y=w1397) -> (x*y=w1398:i16)
          }
        }
      }
    }
    frame Enabled {
    }
  }
  n782 = disable-structure shown="Disabled" {
    disable-tunnel: w4 -> [w1428 _]
    disable-tunnel: w2 -> [w1427 _]
    frame Disabled {
      n783 = while "473 nm blue  fluorescent laser interlacing (DO to blue laser digital control input)." {
        shift-right: [w1432] -> _
        shift-left: w1427 -> [w1437]
        shift-right: [w1431] -> _
        shift-left: w1428 -> [w1429]
        stop <- FALSE stop-if-true
        n784 = flat-sequence {
          tunnel: w1437 -> [w1440]
          tunnel: [w1441] -> w1435
          tunnel: [w1440] -> w1433
          tunnel: [w1439] -> w1430
          tunnel: w1429 -> [w1439]
          tunnel: [w1444] -> w1436
          tunnel: w1435 -> [w1444]
          tunnel: [w1443] -> w1434
          tunnel: w1433 -> [w1443]
          tunnel: w1430 -> [w1442]
          tunnel: [w1453] -> w1432
          tunnel: w1436 -> [w1473]
          tunnel: w1434 -> [w1470]
          tunnel: [w1462] -> w1431
          frame #0 {
            n785 = call "Loop Timer14"("Count(Ticks)"=w1440) -> ("Tick Count(Ticks)"=w1441:u16)
          }
          frame #1 {
            n786 = xnode "FPGA I/O Node"("Connector1/DIO28"=w1442) -> ()  [unwired: 1 in, 1 out]
          }
          frame #2 {
            n787 = feedback-in #66(w1473) -> ()
            n788 = feedback #66(w1473) -> (w1472:u16)
            n789 = Subtract(x=w1473, y=w1472) -> (x-y=w1471:u16)
            n790 = Subtract(x=w1471, y=w1470) -> (x-y=w1446:u16)
            n791 = Number To Boolean Array(number=w1446) -> (Boolean array=w1447:bool[])
            n792 = Or Array Elements(Boolean array=w1447) -> (logical OR=w1445:bool)
            n793 = Boolean To (0,1)(Boolean="+ phase (BI D)") -> (0, 1=w1458:i16)
            n794 = Multiply(x=w1458, y="Phase count adjustment (BI D)") -> (x*y=w1455:i16)
            n795 = Boolean To (0,1)(Boolean=w1445) -> (0, 1=w1452:i16)
            n796 = To Unsigned Byte Integer(number=w1452) -> (unsigned 8bit integer=w1449:u8)
            n797 = feedback #67(i16 0) -> (w1456:i16)
            n798 = feedback #68(u8 0) -> (w1450:u8)
            n799 = Add(x=w1449, y=w1450) -> (x+y=w1448:u8)
            "Blue Late Counter (D)" <- w1448
            n800 = feedback-in #68(w1448) -> ()
            n801 = Subtract(x=w1456, y=w1455) -> (x-y=w1454:i16)
            "BI Relative phase (D)" <- w1454
            n802 = feedback-in #67(w1454) -> ()
            n803 = feedback #69(TRUE) -> (w1465:bool)
            n804 = case shown="2" "Blue Laser Operating Mode (D)" {
              tunnel: [TRUE FALSE w1479] -> w1462
              tunnel: w1465 -> [_ _ w1476]
              frame 0, Default {
              }
              frame 1 {
              }
              frame 2 {
                n805 = Not(x=w1476) -> (.not. x?=w1478:bool)
                n806 = Select(t=w1478, s="Invert BI (D)", f=w1476) -> (s? t:f=w1479:bool)
              }
            }
            n807 = Not(x=w1465) -> (.not. x?=w1461:bool)
            n808 = Select(t="Blue interlace ON count (D)", s=w1461, f="Blue interlace OFF count (D)") -> (s? t:f=w1467:u16)
            n809 = Subtract(x=w1467, y=w1446) -> (x-y=w1459:u16)
            n810 = Add(x=w1459, y=w1455) -> (x+y=w1453:u16)
            n811 = feedback-in #69(w1461) -> ()
          }
        }
      }
    }
    frame Enabled {
    }
  }
